vi "PECT - Scan_time gate_counter - 2.vi"() -> ()   [LabVIEW 2012]
uses:
  <vilib>/DAQmx/read.llb/DAQmx Read (Counter U32 1Chan 1Samp).vi
  <vilib>/DAQmx/read.llb/DAQmx Read (Analog 1D DBL 1Chan NSamp).vi
  <vilib>/DAQmx/read.llb/DAQmx Read (Analog Wfm 1Chan NSamp).vi
  <vilib>/Instr/_visa.llb/VISA Configure Serial Port (Instr).vi
  <vilib>/DAQmx/create/channels.llb/DAQmx Create Channel (AI-Voltage-Basic).vi
  <vilib>/DAQmx/create/channels.llb/DAQmx Create Channel (CI-Count Edges).vi
  <vilib>/DAQmx/configure/timing.llb/DAQmx Timing (Sample Clock).vi
  <vilib>/DAQmx/configure/task.llb/DAQmx Configure Logging (TDMS).vi
  <vilib>/DAQmx/configure/trigger.llb/DAQmx Start Trigger (Digital Edge).vi
  <vilib>/DAQmx/miscellaneous.llb/DAQmx Fill In Error Info.vi
  <vilib>/express/express analysis/Spectral/Block/exnSpectralBlock spectral measurements PSD poly.vi
  <vilib>/express/express analysis/Spectral/Block/exnSpectralBlock spectral measurements PSD WFM.vi
  <vilib>/express/express analysis/Spectral/XNode/ExpressSpectralMeasurementsBlockNode.xnode
  <resource>/objmgr/daqmx.rc
  <vilib>/measure/NI_MABase.lvlib
  <vilib>/Platform/NI_3dgraph.lvlib
  <vilib>/DAQmx/write.llb/DAQmx Write (Analog 1D Wfm NChan NSamp).vi
  Global_data.vi
  <vilib>/DAQmx/create/channels.llb/DAQmx Create Channel (AO-Voltage-Basic).vi
  <vilib>/DAQmx/write.llb/DAQmx Write (Analog Wfm 1Chan NSamp).vi
panel:
  in  "Repair Line Col":bool
  in  "Repair Line Row":bool
  in  "Line Col":dbl=167.0
  in  "Line Row":dbl
  in  "Filter":bool caption="Scan"
  in  "low cutoff freq: fl":dbl=40.0 format="%0.2f"
  in  "Backindex":i32
  in  "Backdata":bool caption="Scan"
  in  "ColorMapAutoScale":bool=TRUE
  in  "Min":dbl=-0.8
  in  "Max":dbl=0.6
  in  "Inverse":bool caption="Scan"
  in  "Odd":bool caption="Scan"
  in  "DiffY":bool caption="Scan"
  in  "DiffX":bool caption="Scan"
  out "Completed":bool
  out "Motor Pulse Count":i32
  in  "Counter Pulse from Motor":tag="Dev6/ctr0"
  in  "Input Counter Terminal":tag="PFI8"
  in  "Open tdms":bool
  in  "Pulse generator":T1={"Waveform Type"=2, "Amplitude"=10.0, "Frequency"=1000.0} {"Frequency" format="%0.2p"; "Amplitude" format="%0.2p"; "Waveform Type" items=["Sine Wave", "Triangle Wave", "Square Wave", "Sawtooth Wave"]}
  out "Cur. X":dbl format="%#_4g"
  out "Old X":dbl
  out "Cur. Y":dbl format="%#_4g"
  out "Old.Y":dbl
  out "Compare X":dbl
  out "compareY":dbl
  out "y >= 0":bool
  out "x >= 0":bool
  out "move X":dbl
  out "move Y":dbl
  out "deltaY":dbl
  out "delta X":dbl
  in  "Move Distance":dbl=5.0
  in  "Emergency Stop":bool
  in  "Stop 3":bool
  in  "Home Y":bool
  in  "Home X":bool
  in  "Back":bool
  in  "Front":bool
  in  "Left":bool
  in  "Right":bool
  in  "Stop Scan":bool
  out "Start Pos. X":dbl=-22.5 format="%#.4f"
  out "Start. Pos.Y":dbl=18.8 format="%#.4f"
  out "열거형":T2(ring)
  out "숫자형":i32
  in  "Gate 2":dbl=50.0
  in  "Gate 1":dbl
  out "No.data":i32
  in  "Save Scan mode":bool caption="Save Process"
  in  "Plot style":i32(ring)=5 items=["cwLine"=1, "cwPoint"=2, "cwLinePoint"=3, "cwHiddenLine"=4, "cwSurface"=5, "cwSurfaceLine"=6, "cwSurfaceNormal"=7, "cwContourLine"=8, "cwSurfaceContour"=9]
  in  "Stop 4":bool
  in  "ViewMode":i32(ring) items=["cwViewXYPlane", "cwViewXZPlane", "cwViewYZPlane", "cwViewUserDefined"]
  in  "Scan":bool
  in  "Open csv":bool
  in  "Tab Control 2":T3(tab)
  out "Hall sensors signal":waveform(dbl)[](graph)=[{"t0"=timestamp(3525645621.636764 s since 1904-01-01), "dt"=1.9999999999999944e-06, "Y"=array[2100 elements], "attributes"=variant("NI_ChannelName"=variant(string "Dev1/ai0"), "NI_UnitDescription"=variant(string "Volts"))}, {"t0"=timestamp(3525645621.636764 s since 1904-01-01), "dt"=1.9999999999999944e-06, "Y"=array[2100 elements], "attributes"=variant("NI_ChannelName"=variant(string "Dev1/ai0"), "NI_UnitDescription"=variant(string "Volts"))}]
  out "Feature Extraction":dbl(graph)=0.021153968958947764
  out "Waveform Graph 2":waveform(dbl)(graph)
  out "Power spectral density":cluster{"f0":dbl, "df":dbl, "magnitude":dbl[]}[](graph)=[{"f0"=0.0, "df"=238.09523809523876, "magnitude"=[-25.4340272409559, -28.495970805276507, -69.09064054555873, -79.11355871279994, -75.69366097931027, -84.18131507822396, -80.50168881348966, -82.72314293089615, -87.19630499623688, -82.83568021481967, -89.95290866002237, -85.90392585035596, -87.41269111550386, -91.40893948681482, -86.69370819914215, -93.36336146616782, -89.019380476413, -89.73232030153878, -94.58261196624535, -89.16287927388944, -94.965890302584, -91.86846413178648, -91.95327957161693, -97.62687167891286, -91.59993648735762, -97.30685711015555, -93.8350762480425, -93.27921214218685, -99.59438563802183, -93.1824258709588, -98.3113125531512, -95.45425138584356, -94.39327135467576, -100.65352961491782, -94.55889081970952, -99.40788907105079, -97.93617495318924, -96.19517579047603, -103.97036797797732, -96.40295202889732, -99.7036956909043, -99.48760137175819, -97.46192979187015, -106.29271483151813, -97.51447379981207, -99.86179280251669, -100.43811038443037, -97.59011642740829, -105.58363666166275, -99.01126121197593, -101.01575323613292, -101.90167607549864, -98.61952569586691, -106.73670466995647, -99.29976101634999, -101.54959604687718, -105.17330050767885, -100.09392305285375, -109.78264848704497, -100.98914236173123, -101.81665207962125, -105.42358374403365, -99.82880728595141, -107.07330885402075, -101.07712607444097, -101.03780825357597, -107.32811151840846, -101.221643458408, -105.63776326231454, -101.8420593566944, -101.80081629073969, -107.47915505307212, -101.12986632760553, -106.84901404755908, -102.73715610491038, -101.51552854007832, -107.28771371003282, -101.3928633472346, -107.44515355816633, -104.89304864643535, -103.1455098860718, -110.19910428997925, -102.73063833081197, -107.57101838377707, -104.90574568581201, -103.72599931018533, -109.97178587260123, -103.24611921258705, -108.36098023558972, -106.6408311450923, -104.73569536588386, -116.21683530762306, -105.02627439976544, -107.15856030450797, -109.81191038702062, -105.53476822084077, -119.10077766590356, -105.31867536160968, -106.9718410299748, -108.34458911268797, -104.70307996109247, -114.76704583683203, -106.29948298493936, -108.55077108437321, -112.16618350190343, -105.98453547558171, -114.68576835450673, -107.50968901677987, -107.89174277914348, -111.59875709602721, -106.69368240333122, -114.93273233954758, -105.23904516482949, -106.00272331017348, -110.36103151258544, -104.93177986717492, -110.8835476773746, -106.69346348818806, -106.66103973993782, -119.11729839814336, -108.06338160849775, -114.5879267769655, -108.59816838472844, -107.53189260743514, -114.07390818184973, -106.70996756049796, -113.27381274118753, -109.50270539577696, -107.37282420343303, -113.4779718725949, -106.04267666963091, -111.30294425571472, -112.46717993668915, -109.13164915488709, -116.65287200885172, -107.03002573045511, -110.21479040603631, -112.476075561056, -106.97710947409149, -119.42145279296255, -108.3200486628316, -110.46641858585929, -117.16650627564961, -109.73297826697552, -120.31689830731365, -107.19513745371916, -110.66663569403087, -113.30365980039964, -110.01971553524372, -123.68660617105166, -110.8171755739396, -111.11382172813546, -117.76239209582961, -109.49899370205401, -115.22252846498625, -111.1932077339224, -112.38235939086871, -118.22207022901702, -110.6546796895719, -116.97450780644367, -110.82401674194465, -111.96705198878843, -118.28092956599232, -110.5621503678909, -121.25720613496851, -111.98371482341479, -113.27928013246557, -111.96833712758355, -108.56859286664552, -120.32790468431601, -110.82699792221703, -110.79062667340345, -122.65756767769517, -110.48843456045427, -116.8782055296399, -115.43719816168479, -114.47619780315773, -121.42183196132746, -111.60631415727042, -120.68077308056417, -109.35478690141552, -109.03210709352732, -120.6260555904793, -109.47936424950136, -113.33719701518146, -112.88325992990137, -110.99901978536154, -123.19636626521421, -109.09861317900774, -113.33125158106256, -115.35673297389727, -112.77249677632989, -124.61163141716472, -114.68140920359865, -121.89642913325117, -115.47413298424323, -112.82196063671608, -127.87542521315149, -111.54178118788309, -113.6448752704395, -120.76569423868874, -112.98651214877823, -123.18868565400437, -115.41399838634062, -115.46853076016815, -116.40989072804102, -110.69611347288615, -132.23164080331392, -114.76376391429793, -121.7246597336247, -117.46893009589195, -114.01899156779395, -125.22079066032327, -114.59524199183258, -114.50034890537415, -122.9532092227648, -113.72727798159212, -125.65163915514907, -113.4793801211504, -110.4090756414644, -125.63592649005872, -114.22938378193007, -116.74947251106808, -121.60535557984142, -116.79385283402802, -122.44667696630361, -113.43873413563811, -123.28159708694415, -113.92892974938164, -114.01193823589753, -121.62751955742443, -118.76839573694522, -125.52998605097204, -115.19609643487229, -117.49409595176479, -117.08423885198002, -119.48314867245172, -125.01675515413412, -117.92668164142911, -115.55962389856793, -125.63488616674975, -119.11862859365166, -114.78860770332909, -117.18339781294443, -111.18063004722558, -118.31775966044624, -111.6867367949252, -114.57226159377, -119.36541212960576, -113.90245139442648, -132.46343443313128, -120.1282759002165, -121.05279009698619, -118.9115822659523, -121.23280439248342, -116.31914159559688, -127.38829313950257, -117.34673005740623, -115.95249861902771, -114.9301657394146, -123.22361802797445, -110.83274939062106, -116.16624248562111, -116.76753364192771, -113.94454545069023, -122.95736945775944, -118.66755800656253, -129.1462641201204, -116.6351050110328, -117.22529407303742, -123.80212197360244, -115.89792176423389, -114.25823938606595, -125.60467961977515, -114.59958849364433, -121.70071005514421, -118.25968972451209, -114.69929400946009, -123.88209034116528, -115.03869272537257, -117.52034211782204, -115.27990843516797, -117.85366603932033, -125.16865559622727, -118.21960424638507, -119.69008755413566, -117.24640963460672, -114.32867295013791, -119.1576982419508, -122.85495988425586, -116.3373010103401, -114.53730203699834, -115.67017599990201, -127.144321037601, -115.73849102686786, -117.7626163106355, -119.7346592991025, -117.41317517684553, -125.0417974461613, -114.5488949833583, -116.59812516173781, -119.91064563147799, -115.27933218667663, -122.09990513751134, -120.95678574143693, -123.25641714743752, -112.5173710452192, -113.53735878806998, -129.23914933506734, -116.27157269711533, -148.4020512032711, -118.84888216023774, -123.82550527215588, -116.87770979616658, -111.32191810025745, -124.32675905891588, -114.37182733794062, -121.10713785851372, -122.59698730059695, -116.38346694563282, -121.69144349152856, -119.00883142493832, -110.81886738196273, -120.7909830607913, -115.01780448665316, -114.52055121633796, -132.6824191654361, -116.330695115645, -126.4664151018508, -118.32717907779282, -118.7288071595281, -120.42749846140066, -112.53185615773879, -124.26026008984286, -114.24089252048742, -120.00368190003405, -114.71738500842926, -112.92262025927133, -129.21127897188563, -113.5947811765517, -117.80802009651353, -117.0133790103226, -112.19210322760304, -118.17549968071762, -119.3256187825503, -118.84981507334446, -121.39118969751144, -114.64543555194373, -119.84814933224528, -114.09123407848944, -116.22899352170892, -116.41650104077173, -113.70057202673476, -124.52773908304957, -114.87372641784933, -116.11651108221098, -121.68680962246994, -115.78306007961302, -122.22621008657796, -118.81157995182392, -113.9402115821658, -132.636729517989, -114.49554876936634, -119.50980190398928, -123.27410972236837, -118.52851881066383, -122.25212982572599, -117.13947036230024, -120.85005588797962, -118.41526503460501, -117.61788553858068, -126.3872056783977, -114.98198608543298, -119.7789938911847, -120.84873579392627, -114.38831474301695, -153.35954756825245, -113.19505610638078, -114.17454820985151, -127.41069917723112, -114.92677241657191, -125.49053973810628, -113.36382196587914, -119.96785250843519, -122.47388530423243, -116.38671253508838, -120.0905790211523, -119.83326265062107, -117.88168146696918, -122.3132169880757, -115.87324909105399, -125.92003267803432, -113.96860176867415, -114.49156118371398, -127.52634390035722, -115.05967156528004, -126.82020221981517, -117.93643187259194, -116.51163213641807, -119.47551219110167, -119.55225172256931, -116.9512257852571, -122.23153124485954, -120.8368476753637, -121.48473913072222, -115.83122660909913, -135.74260014140523, -116.58358375805423, -118.15236945484727, -119.06674062398864, -115.7844834762477, -125.06111738611818, -114.7801535050972, -115.2696605691888, -123.98656374010793, -119.29025555731172, -118.29146803784099, -119.55696172158135, -118.06884171238352, -127.81587648134607, -120.41730580797976, -123.49626136731604, -112.2147141798107, -116.22555232584983, -132.79419178871254, -119.66964883124663, -117.20946469243259, -118.20939292735417, -115.6951914646649, -129.64892855822356, -114.27056999288617, -120.31005512957381, -117.41846777372632, -115.50158386260813, -124.69777160737624, -115.2892897247205, -123.61522771666871, -113.75248734362687, -113.22999749252833, -129.3490509395313, -116.88137735661701, -116.94110280242681, -119.50244079984806, -119.30521139999144, -128.17199984115797, -118.06736594940236, -116.05331575995922, -121.29670750650897, -116.1140297602044, -125.090619084802, -121.41807296062154, -120.01332757902264, -120.54914530643151, -116.49738633175463, -122.32551291835904, -118.3190808346865, -118.92638453656723, -122.48819531011718, -117.01021725424317, -120.98896352560598, -117.23831688685218, -121.27915259197124, -121.20017251921661, -117.6155648860373, -120.91300272912063, -117.94438460863424, -115.94437430101533, -123.35904829443987, -117.74011174503076, -121.54935745388448, -120.82564553545025, -121.98951430455743, -120.24858103448778, -116.44403527138395, -112.79571494351876, -112.42801913096545, -110.1697573019791, -115.34500457736401, -119.81921052956707, -129.82600951154313, -115.5862301263047, -112.59292882433087, -120.79009137478283, -131.32849293387295, -113.61194478398238, -123.48568856527031, -119.17507777781304, -123.09261867490484, -116.97755217417308, -123.94453461434183, -116.58080525616379, -119.64289646280756, -122.90202645580743, -126.66219093058154, -121.95048829056148, -115.72578023509817, -116.70117814464484, -121.91050280869723, -118.25299095698178, -116.45905559047064, -132.57794493731578, -121.65327820443292, -120.9816664775787, -117.17270262269045, -120.27433984830965, -125.89418976028173, -119.09563505847817, -126.9693215534833, -113.17465524665704, -118.98702092883116, -119.83822568580342, -120.45832738089722, -120.67735960513633, -127.38676010839353, -127.65777338183055, -118.37446329057411, -115.61355494839711, -119.94568688114103, -116.06619937633681, -126.348857777089, -118.92850079147068, -119.5416617639739, -132.47075644221843, -118.08809356028496, -123.16186463092723, -121.51579486791232, -122.88983670053283, -129.5195538417256, -120.4730389608841, -132.16486858341602, -122.34690358436781, -120.71922104337597, -114.29260860841114, -117.67902631803368, -124.7040155514909, -123.51274592117205, -120.02297921674332, -136.54655493811157, -120.45629227407751, -119.06410204276258, -127.91681714792554, -122.82090055753153, -125.16838176650813, -121.79565386970478, -119.79607311590995, -126.54861375039647, -121.59135878113302, -132.8348640697562, -118.1305434733294, -120.46070148841905, -122.69571910896963, -117.6534954653865, -124.15742546824006, -120.73646926947502, -124.82696993800742, -124.513836786494, -123.15395713389651, -124.62395468806395, -117.21365768658171, -119.32635871968456, -121.48532284413152, -119.38242892643675, -126.25575652510352, -123.27133124029851, -117.58533922728374, -118.17710108929799, -114.99496360200965, -117.77133194647278, -111.34898201101595, -111.50817058307922, -119.0703124690998, -127.70676079885351, -121.8704969141074, -125.93154214283446, -118.65628450081473, -122.47918878348962, -117.9651589546518, -126.13560583004508, -122.42294805637847, -133.924453763793, -117.2082573038767, -117.6525335446734, -122.92077297426977, -122.04624645756786, -116.43289028226238, -117.93180959338378, -129.02356734231915, -117.95493621286326, -120.7555929766252, -120.76782849311112, -123.06287498470708, -117.83798593857965, -123.43423215434719, -120.15190119516652, -120.48240443128407, -143.29738987393452, -123.46572247444769, -120.89055325172792, -125.66715973809033, -118.26887578998644, -117.01836200028421, -121.33021830755509, -119.68846363313813, -122.60689066103069, -116.26858138914181, -119.59360791972998, -122.94866175463353, -114.174409515556, -118.00516930888391, -121.56978543579633, -135.87799017759036, -117.50816594504829, -122.82539428457626, -123.82103443155845, -124.77975840345442, -121.13340798086698, -120.93607435603558, -133.15787160745222, -120.70545628137863, -125.02155972441679, -122.04666465472178, -118.01234649746348, -127.88767491042842, -119.02096620167217, -120.16031065152875, -122.25406107859625, -121.72733059051095, -120.61357375519918, -118.63962847172827, -134.3857741605498, -116.3600853185034, -117.26695700691671, -119.9176982185873, -113.45576465218444, -126.69779573632724, -114.39554522802246, -116.8457146515868, -116.34219889483086, -119.30011291548334, -120.01163291843496, -114.29497178248809, -127.65687642749229, -119.58556923753022, -129.8593054181261, -122.2353645100479, -120.79536520223796, -119.83284028355028, -117.7991246185715, -128.390292904734, -119.78079925213122, -125.478913448993, -113.89747777944768, -112.66620124153357, -124.3475049842711, -120.85847303094337, -132.91807981902295, -119.523494985723, -116.65149909866443, -119.73287290436721, -127.63237851524192, -127.23413304048789, -120.87585453904362, -121.08540368080186, -134.91071939669257, -117.75375801669338, -117.2683014590723, -120.9739099492833, -118.23809733632451, -120.94065804928206, -123.88077510875804, -118.13812819300607, -122.60294123365466, -126.97075898006995, -120.18754789731035, -124.71238663441227, -120.55456557278582, -130.94599087480253, -111.18288669417035, -112.27708791831247, -126.0512034600378, -117.41881712783596, -128.20553880273903, -117.29482600885808, -118.2045526390752, -127.81966672699878, -117.03716165902529, -115.46711739757512, -117.15363929234843, -121.87599671671335, -121.19736800869221, -126.5301786755875, -131.20754947382918, -124.40138004810741, -129.0562496906515, -121.06816554587536, -121.01023627802867, -138.6137911215848, -120.12495002524031, -121.38510517514229, -122.79804220535513, -116.97501378195477, -118.82011581137473, -114.0229185604644, -119.54287501990726, -114.64474566771625, -117.76935669872461, -123.81082574158907, -118.51678358865587, -128.9664755188374, -123.45357998434133, -122.74888841574231, -120.74640581234044, -126.956344345126, -119.95682140104577, -118.8873101779055, -124.41062359284174, -128.97304498664363, -123.86287113204068, -127.30257087528216, -120.61364220528216, -114.45119129304715, -119.68384044686806, -131.29639185291157, -122.31250766293485, -119.57420865241102, -124.74014026002448, -124.87593035709094, -118.4566565612952, -123.76236085976001, -120.84780538841838, -117.68987599773281, -135.06195695255914, -122.56143585795171, -129.04610316842883, -118.32313199570537, -117.77093802786419, -124.46572845786741, -129.1123298336903, -120.88470269965448, -116.69988985752187, -116.84054667499878, -133.76883696987278, -122.32434984927302, -124.98940594457933, -122.56515592789917, -118.31562562243366, -133.97049179545627, -122.33220627999802, -131.16753675316977, -124.69828063969263, -116.37621154460467, -126.1833423168025, -129.62937634161355, -118.46241371150788, -117.52851478852457, -125.32425037236442, -119.0327364293772, -124.2861355894013, -123.24573502278234, -125.52155812053758, -113.75743410709823, -114.79513162658353, -128.58142362588052, -122.48277095196701, -118.94747544412269, -123.86988127835491, -124.78140456983323, -121.53998481875398, -116.01432822539552, -119.20174681160661, -122.75167725800814, -120.58657749420254, -118.51141061842183, -119.24457006171983, -131.43641234223372, -116.00759139055087, -121.24442216102587, -123.29371279953725, -117.608355420454, -116.33684374617326, -118.06291688281922, -121.88761866022774, -121.54820313120047, -119.5051369873635, -126.56611158390913, -118.84012713615805, -121.09285296522563, -124.67955377692547, -147.31451139022337, -116.80660421066897, -114.8367853755961, -120.41026468628925, -123.65666101895222, -119.64837119787269, -116.77480172559095, -116.54263359173909, -124.75286620868079, -117.33721912698883, -116.51795620907136, -118.50086748176733, -128.10381328920522, -122.78098994574157, -120.24716756092855, -119.52743204722819, -115.00407387659232, -108.2853711552629, -108.61086943894702, -119.6228894146785, -124.11132022420912, -125.6202218409766, -123.1749360787656, -118.1971196161698, -123.95075368058998, -121.72140109898365, -123.27106899042522, -123.73035629887062, -121.24369679109273, -121.07381526465288, -113.13965659723667, -118.330755475899, -118.40249076804484, -111.59630598649044, -116.1569506845575, -125.67326089915758, -125.85723567111906, -119.24293277595024, -117.87067617433537, -120.70936924059559, -131.8090588468898, -132.98711569625004, -123.63274249467587, -122.75476917502559, -126.12873814250243, -120.53144270605179, -129.07030822919336, -122.7889410422919, -124.35405971166259, -119.63968579420454, -139.0154441054289, -129.47962001806934, -121.86548015410847, -128.6818469257012, -121.40195873232601, -138.64231053781285, -124.22025721762265, -124.06073958736941, -126.71929802352521, -131.7498459276443, -120.68144109742178, -122.6325588818875, -126.80796617875095, -124.92487955227033, -136.94498040498806, -124.26704334219014, -123.21376211221711, -140.25352033075964, -129.53222319772195, -122.58541579060463, -122.1996729592375, -125.66642108013673, -125.66310429236694, -120.09682773706965, -125.27326633941439, -121.55721878725502, -121.22507119941083, -121.53716878624485, -136.20685498111987, -128.15260146013156, -120.03473972471616, -124.60755958763912, -124.73082500077143, -123.93425949983688, -131.04483249265184, -121.7957035014449, -127.09321441816094, -133.6144579272493, -124.69014595896968, -130.4902091211609, -121.18031440773905, -128.00033943961677, -125.88991118115149, -118.865310745079, -123.69668867733147, -117.98756965862728, -114.40013091842827, -118.28685032521078, -122.23464196869948, -124.8440422629961, -129.66281606870848, -119.440534215621, -124.54391783563877, -124.93447967158188, -121.7258558761523, -122.28817885403082, -127.06889620458577, -128.92172974939206, -120.62932166634072, -126.06847321900452, -123.31471168429935, -121.80350826545656, -129.2574604322076, -125.67225933193998, -125.7801671825605, -129.53804733161627, -119.56756644124712, -128.82490314699373, -124.7689736295626, -120.50019729114693, -124.50603158563972, -122.8120627011088, -125.60528875555717, -123.8817354922713, -124.05570537836674, -120.94568834491936, -118.06056028605255, -124.24390361274648, -125.5716703018188, -127.71949519914061, -130.7001652968252, -126.27701412017494, -133.76810134709916, -128.4738939614179, -120.302550881701, -118.91298143662928, -124.9077318110765, -127.16253699189492, -118.11405934812818, -117.52028071290711, -140.95620572748925, -123.61977932545628, -131.0334379970501, -125.88948384968432, -127.81552331993379, -121.92316280719056, -119.05911238768732, -126.83773251459189, -123.52627415002164, -120.8779561023192, -123.66683567603742, -131.64300993967345, -123.62895847772963, -116.89792951363142, -120.1068259250195, -117.92484706459337, -115.58208487778379, -120.76803581628594, -123.95408562090736, -122.79456549632754, -134.5305398779298, -123.57040300991032, -128.40634159414552, -123.70102187824159, -118.24970739397313, -119.66483900349026, -127.78024313111393, -120.3547204111785, -125.49305364308705, -119.49505591004302, -120.50920386196539, -119.03509516851003, -114.24667300009652, -121.60538636584391, -119.95304417598024, -122.24585853682832, -128.63653016912684, -116.04810628805795, -121.94159862131235, -122.59928204398939, -121.4532410501923, -128.6511474663462, -130.83715595958148, -121.71998300574741, -116.91426629511156, -113.587592058512, -115.59736707638731, -124.65300822631244, -133.32538684258748, -124.02289142873636, -121.54278890993639, -119.02596809402394, -108.90572887117857, -112.14974069608851, -129.21149299565423, -118.82148342951197, -116.65510894288538, -118.39609618084175, -116.53502642884725, -122.47549439965209, -122.23125657046063, -123.68081343116663, -120.67915071600007, -123.6899360128769, -118.56721985209728, -118.36641581191942, -126.96724630704657, -119.36877661672403, -123.07698921198843, -117.80772421906035, -122.82545076270567, -118.82755071380888, -117.21030132539394, -129.760567864525, -118.0816708063509, -125.80573274113647, -121.18434666182338, -121.80987210832065, -130.99259828357094, -125.47223579895922, -123.86818606677002, -118.7118158196511, -119.27778317338742, -127.27333258839096, -119.90672352079164, -140.78772370844268, -118.08251080057329, -119.86636232122572, -118.69482489738232, -119.19106512767372, -123.70988914879189, -121.92566832147995, -123.41378261726373, -120.1715186070818, -117.9079629421116, -117.41960207545632, -123.72833996166874, -127.24377206607298, -124.99098647980887, -129.48803701799955, -129.92351350561592, -120.79284154834647, -119.29601975194524, -136.17244775530037, -126.73975437546255, -128.84068276143336, -125.66374985701982, -136.69026010435715, -125.44409235146617, -119.28138070315057, -118.65017329869724, -118.02521532826772, -122.23736063759657, -121.27846943548622, -116.69850478126861, -119.7711336696722, -123.70776561180185, -118.43344549561263, -123.92390877157247, -117.19637143066551, -117.64112988205311, -127.78399195238529]}, ...(2 in all)]
  in  "3D Surface":refnum<k7>(container)
  out "Record path":path caption="selected path"
  out "Feature extraction scan":dbl[](graph)
  in  "Tab Control":T4(tab)
  in  "Step X":dbl=0.1
  out "Move X":bool
  in  "Direction (+)":bool=TRUE
  in  "Step Y":dbl=0.1
  in  "Y-length":dbl=10.0
  in  "X-length":dbl=5.0
  in  "Save Speed":bool
  in  "Cur. Pos Y":dbl=18.8 format="%#.4f"
  in  "Cur. Pos X":dbl=-22.5 format="%#.4f"
  in  "Travel per Pulse (mm)":dbl=0.002
  in  "2 Rate":dbl=0.2
  in  "1 Rate":dbl=0.2
  in  "2 Min":dbl=1.0
  in  "1  Max":dbl=8.0
  in  "2 Max":dbl=8.0
  in  "1 Min":dbl=1.0
  in  "Parity":u16(ring) items=["None", "Odd", "Even", "Mark", "Space"]
  in  "stop bits":u16(ring)=10 items=["1.0"=10, "1.5"=15, "2.0"=20]
  in  "Data bits":u16=8 min=5 max=8 step=1
  in  "Baud Rate":u32=9600
  in  "COM Port":refnum<visa-resource-name>="COM12"
  out "No. X":i32
  out "No. Y":i32
  out "Sample per Channel AI":dbl
  out "Sample per Channel AO":dbl
  in  "Pulser Cycles":i32=10
  in  "Logging Mode":i32(ring)=10231 items=["Off"=10231, "Log and Read"=15842]
  out "Actual Sample Rate":dbl=500000.0 format="%0.2f"
  in  "Physical Channel":tag="Dev6/ai0"
  in  "Min Voltage":dbl=-10.0
  in  "Max Voltage":dbl=10.0
  in  "Terminal Configuration":i32(ring)=10083 items=["default"=-1, "RSE"=10083, "NRSE"=10078, "Differential"=10106, "Pseudodifferential"=12529]
  in  "Sample Clock Source 2":tag="OnboardClock"
  in  "Sample Rate":dbl=450000.0
  in  "TDMS File Path":path
  out "Actual Sample Rate 2":dbl=800000.0 format="%0.2f"
  in  "Physical Channel(s)":tag="Dev6/ao1"
  in  "Min Voltage 2":dbl=-10.0
  in  "Max Voltage 2":dbl=10.0
  in  "Sample Clock Source":tag="OnboardClock"
  in  "Sample Rate 2":dbl=800000.0
  in  "Offset":bool
  in  "2 Plots":bool
  in  "Edge":i32(ring)=10280 items=["Rising"=10280, "Falling"=10171]
  in  "Pulser Trigger Source":tag="/Dev6/PFI0"
  in  "Duty cycle %":dbl=50.0 format="%#.2f"
  # "Pulse Shape"
  # "Trigger Settings"
  # "Data Processing"
  # "Time gate = %T/2"
  # "Pulse"
  # "Hall Sensors Signal"
  # "Feature Extraction"
  # "Power Spectal Density"
  # "COM  Setting"
  # "Speed  Setting"
  # "Scan  Setting"
  # "Pulse  Channel"
  # "Pulse  Timming"
  # "Sensor  Channel"
  # "DAQ Timming"
  # "Logging Settings"
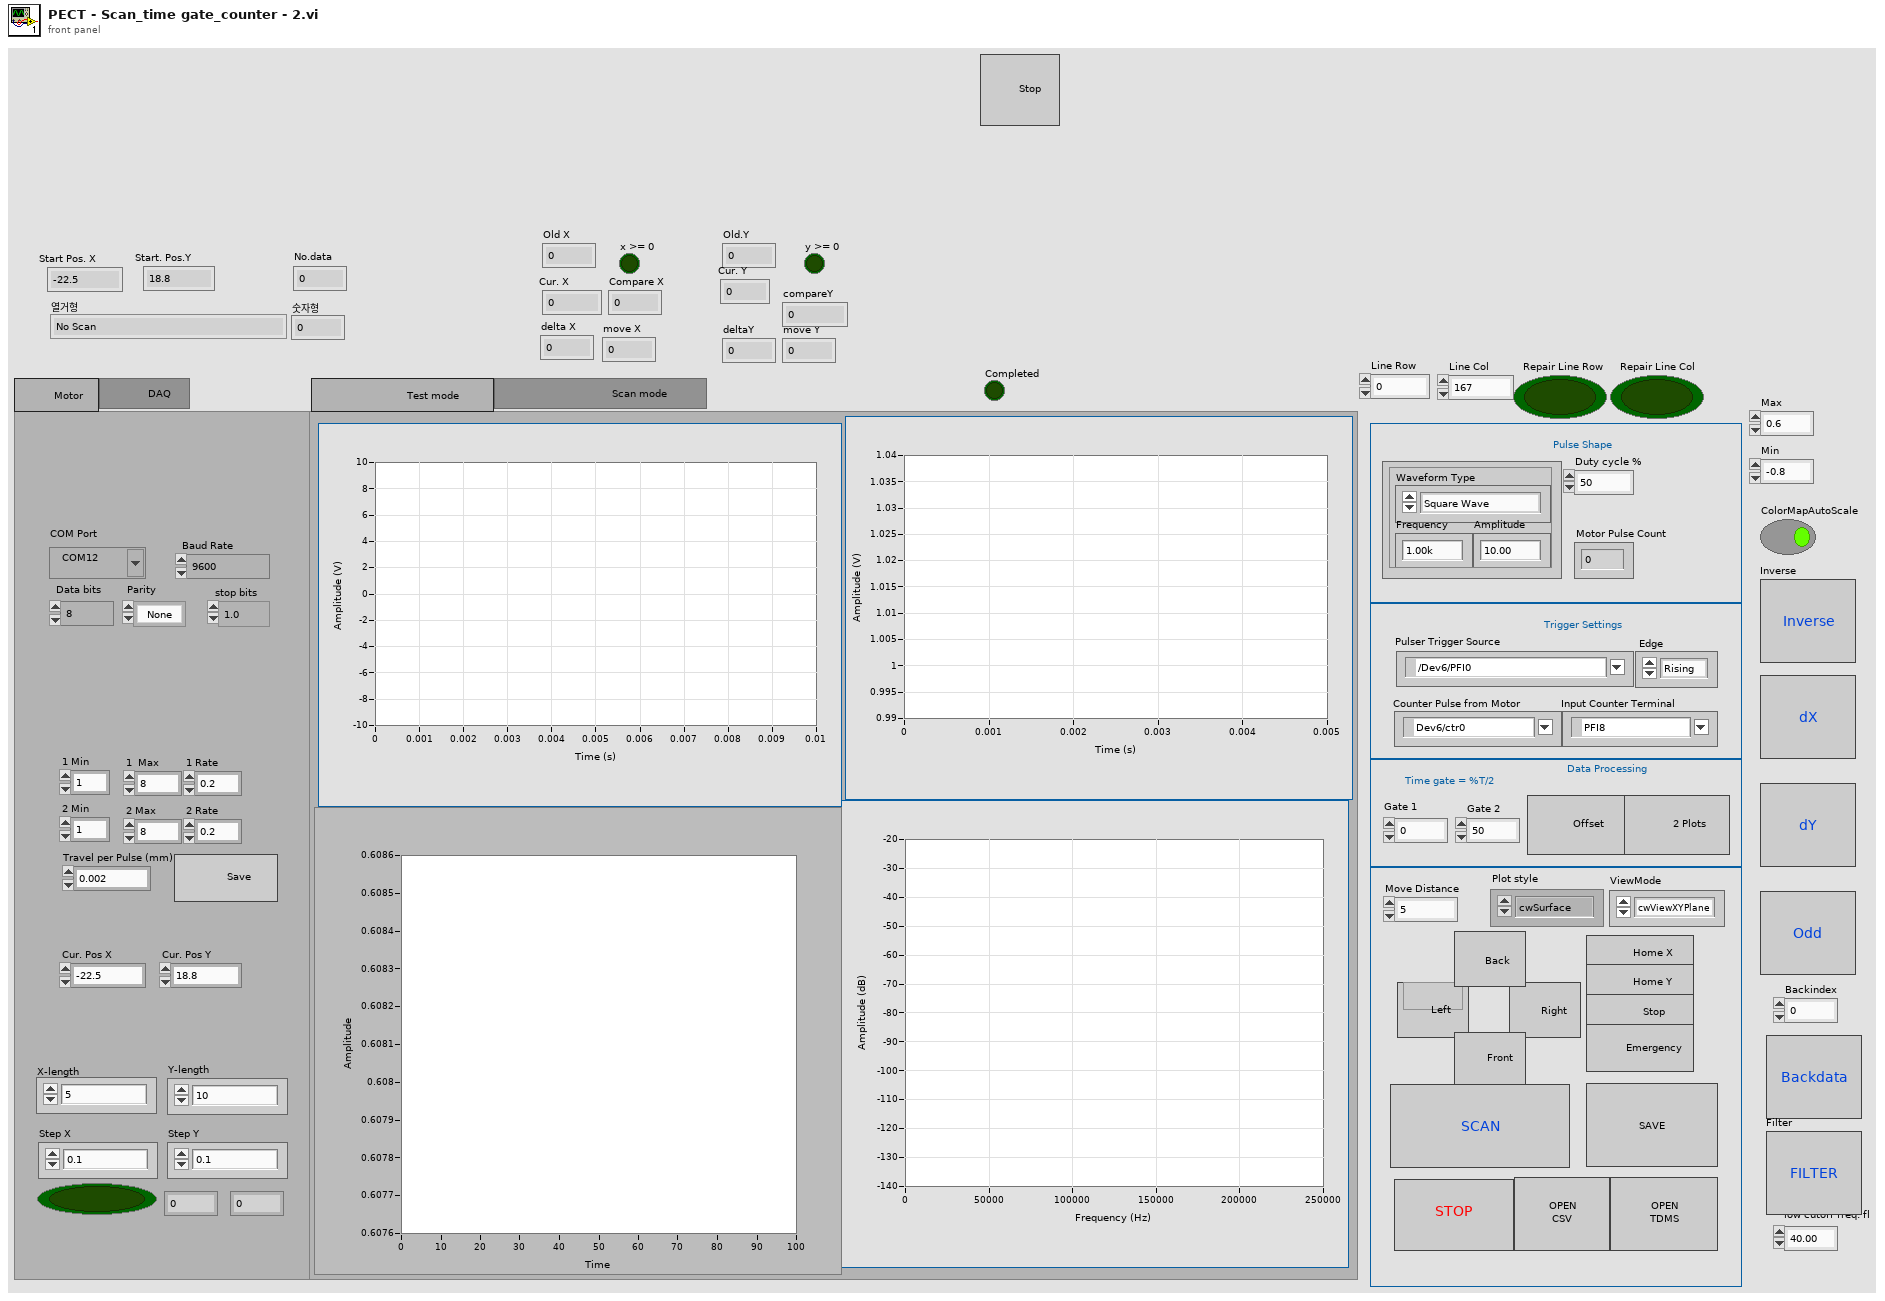
[diagram p1: front panel]
types:
  T1 = cluster{"Waveform Type":u16, "Amplitude":dbl, "Frequency":dbl}
  T2 = enum16{"No Scan", "Move X", "Wait to destination X", "Move Y", "Wait to destinatioin Y"}
  T3 = enum32{"                    Test mode                   ", "                          Scan mode                      "}
  T4 = enum32{"        Motor      ", "          DAQ        "}
  T5 = enum16{"open", "open or create", "create or replace", "create", "open (read-only)"}
  T6 = cluster{"averaging mode":u16, "weighting mode":u16, "number of averages":u32}
  T7 = cluster{"dB On (F)":bool, "unwrap phase (F)":bool, "convert to degree (F)":bool}
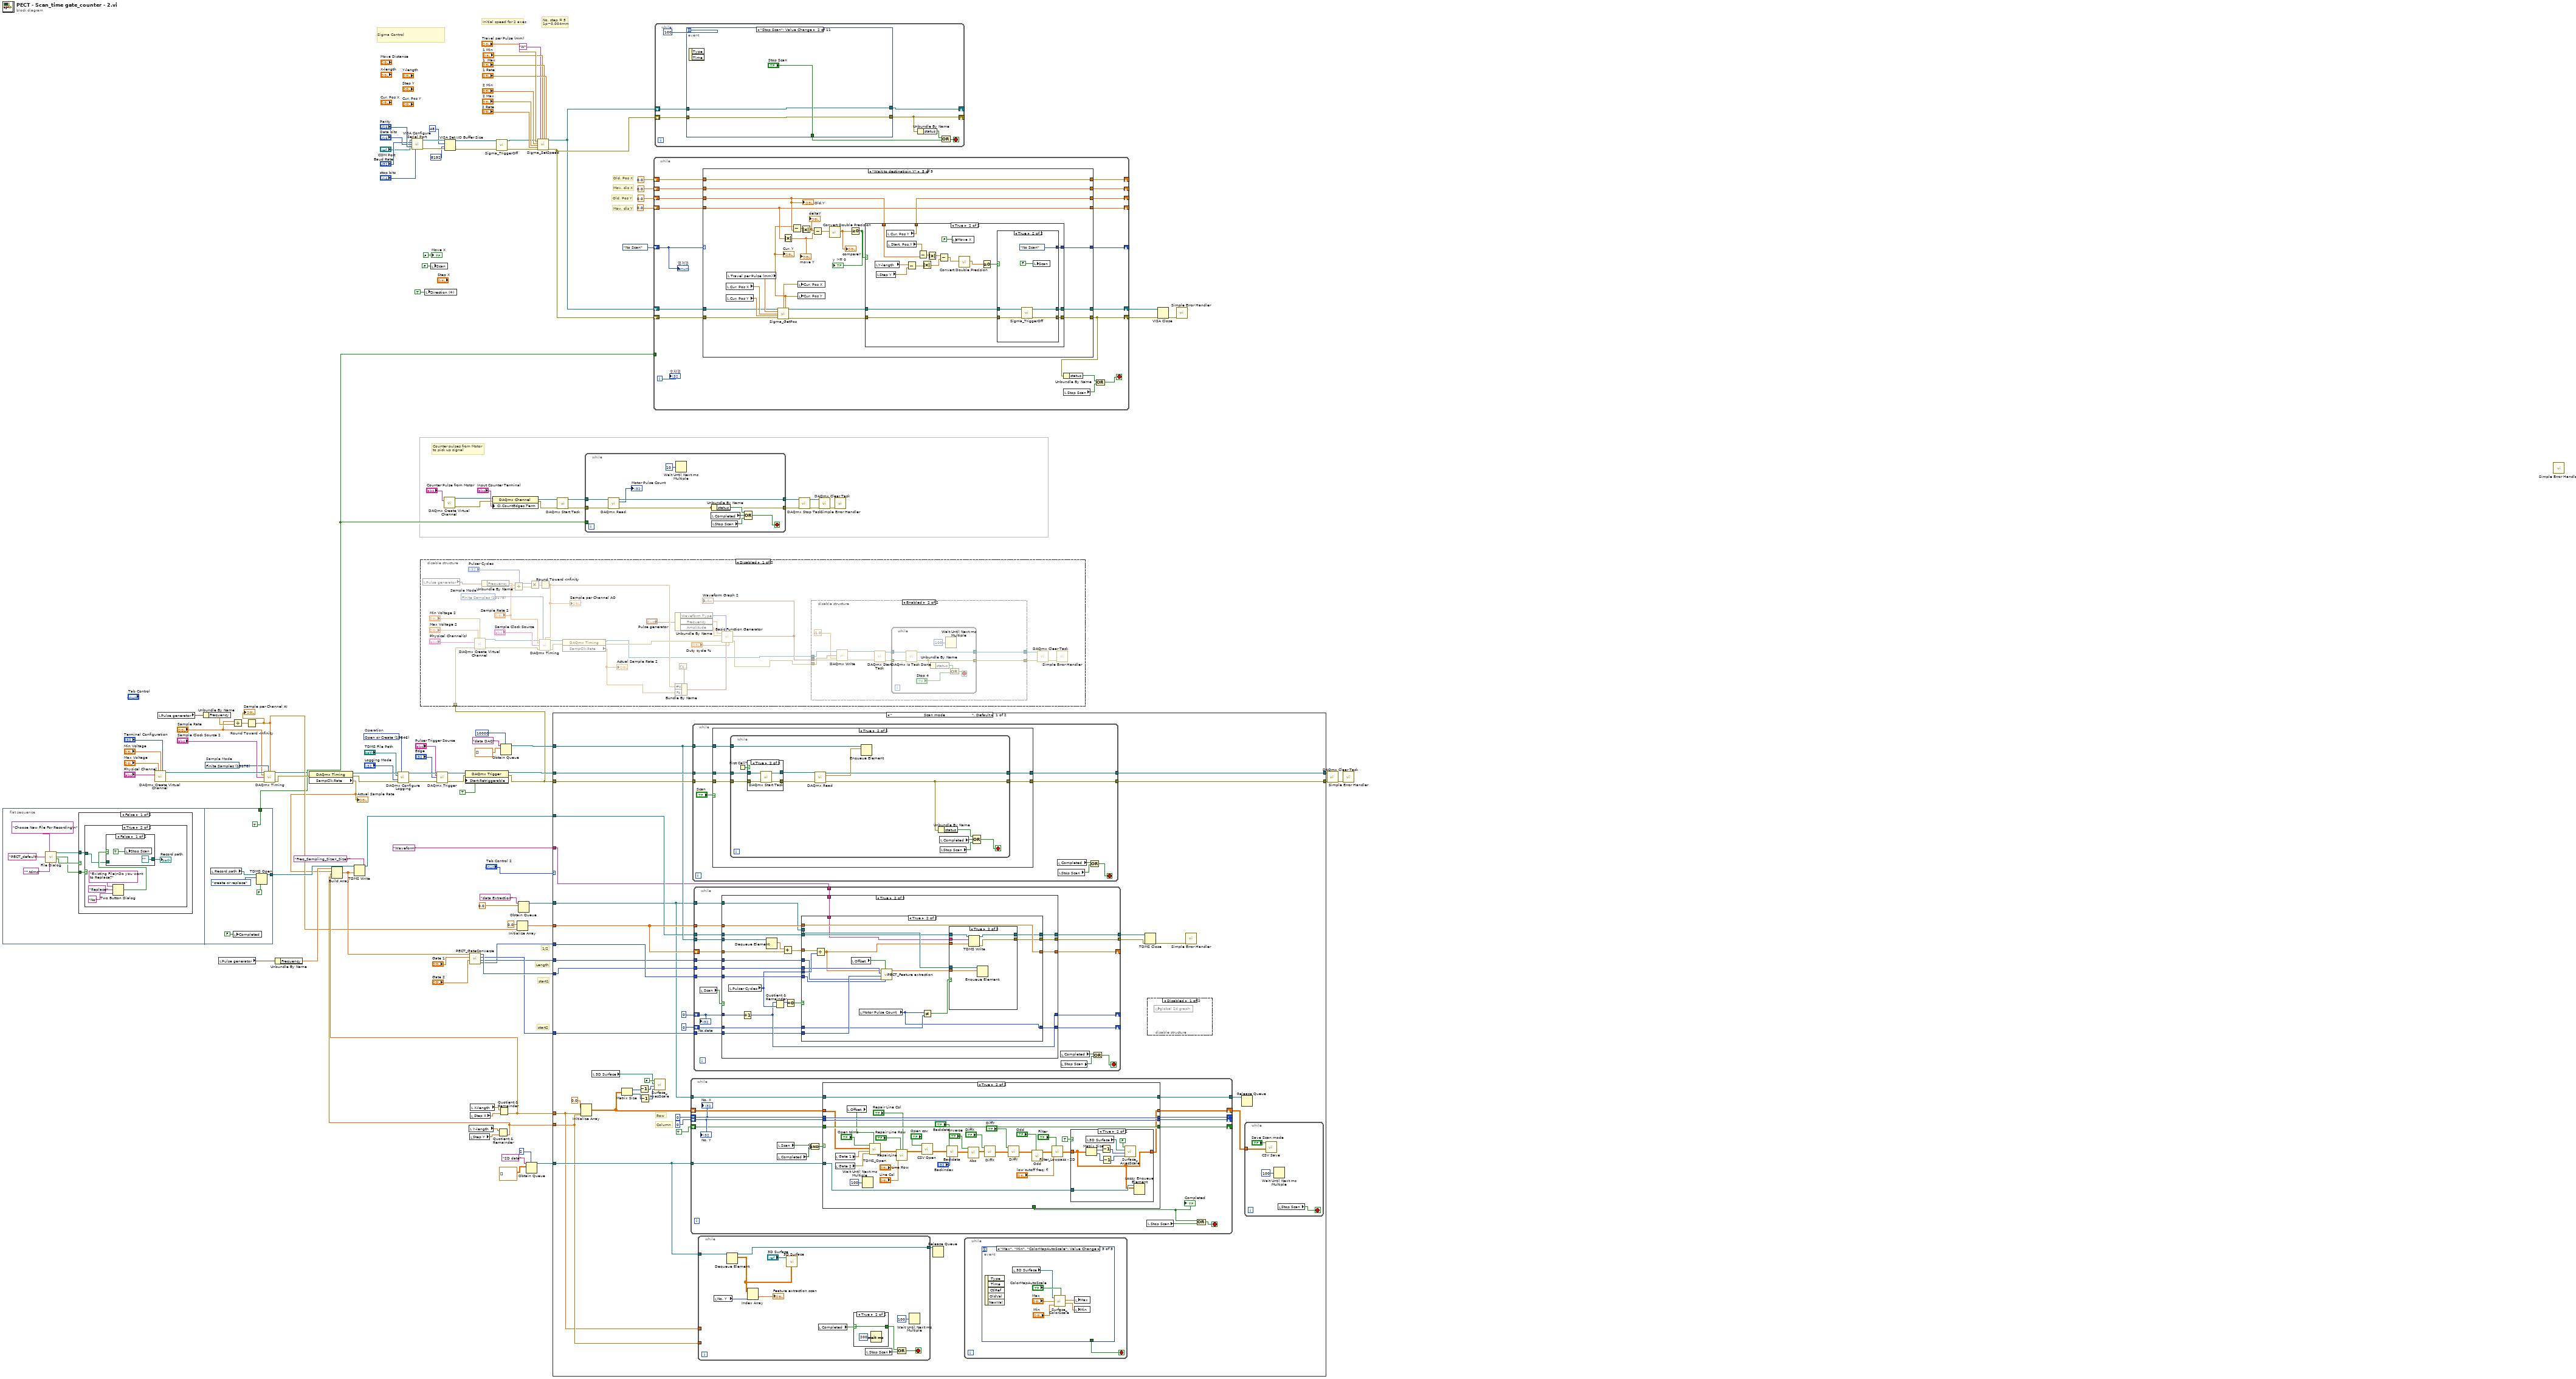
[diagram p0: block diagram]
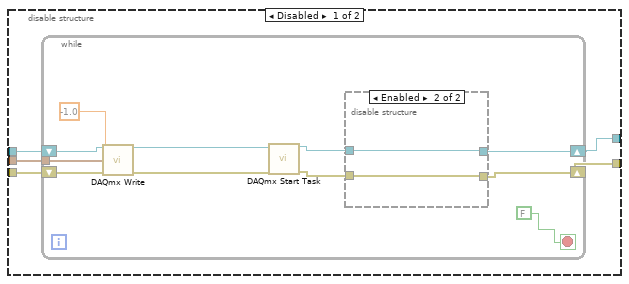
[diagram p2: hidden frame]
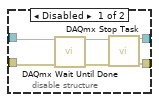
[diagram p3: hidden frame]
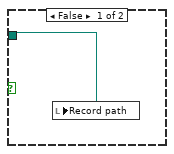
[diagram p5: hidden frame]
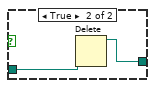
[diagram p6: hidden frame]
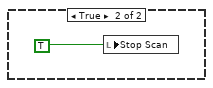
[diagram p7: hidden frame]
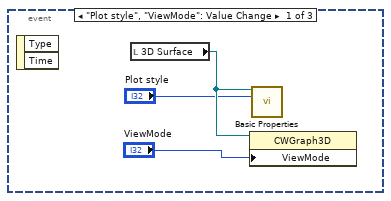
[diagram p8: hidden frame]
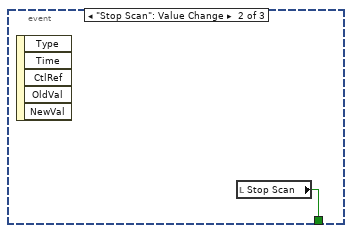
[diagram p9: hidden frame]
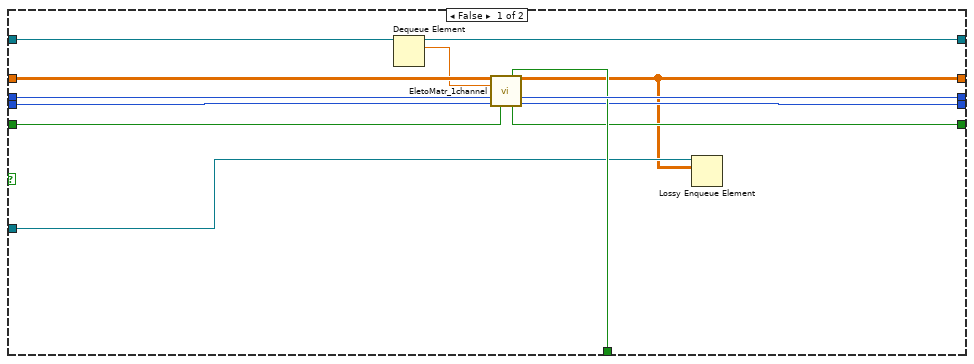
[diagram p12: hidden frame]
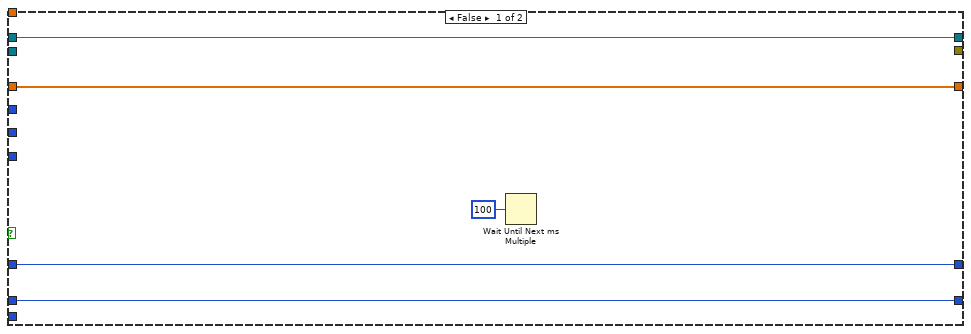
[diagram p16: hidden frame]
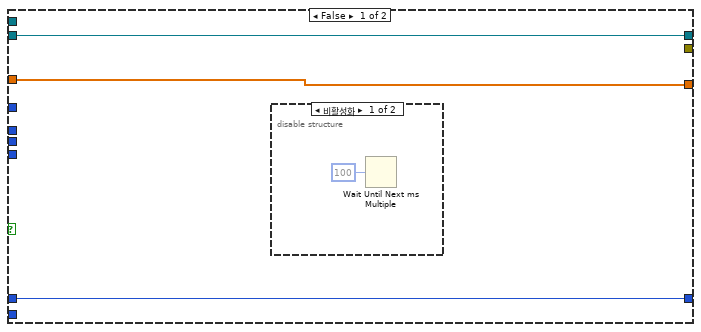
[diagram p17: hidden frame]
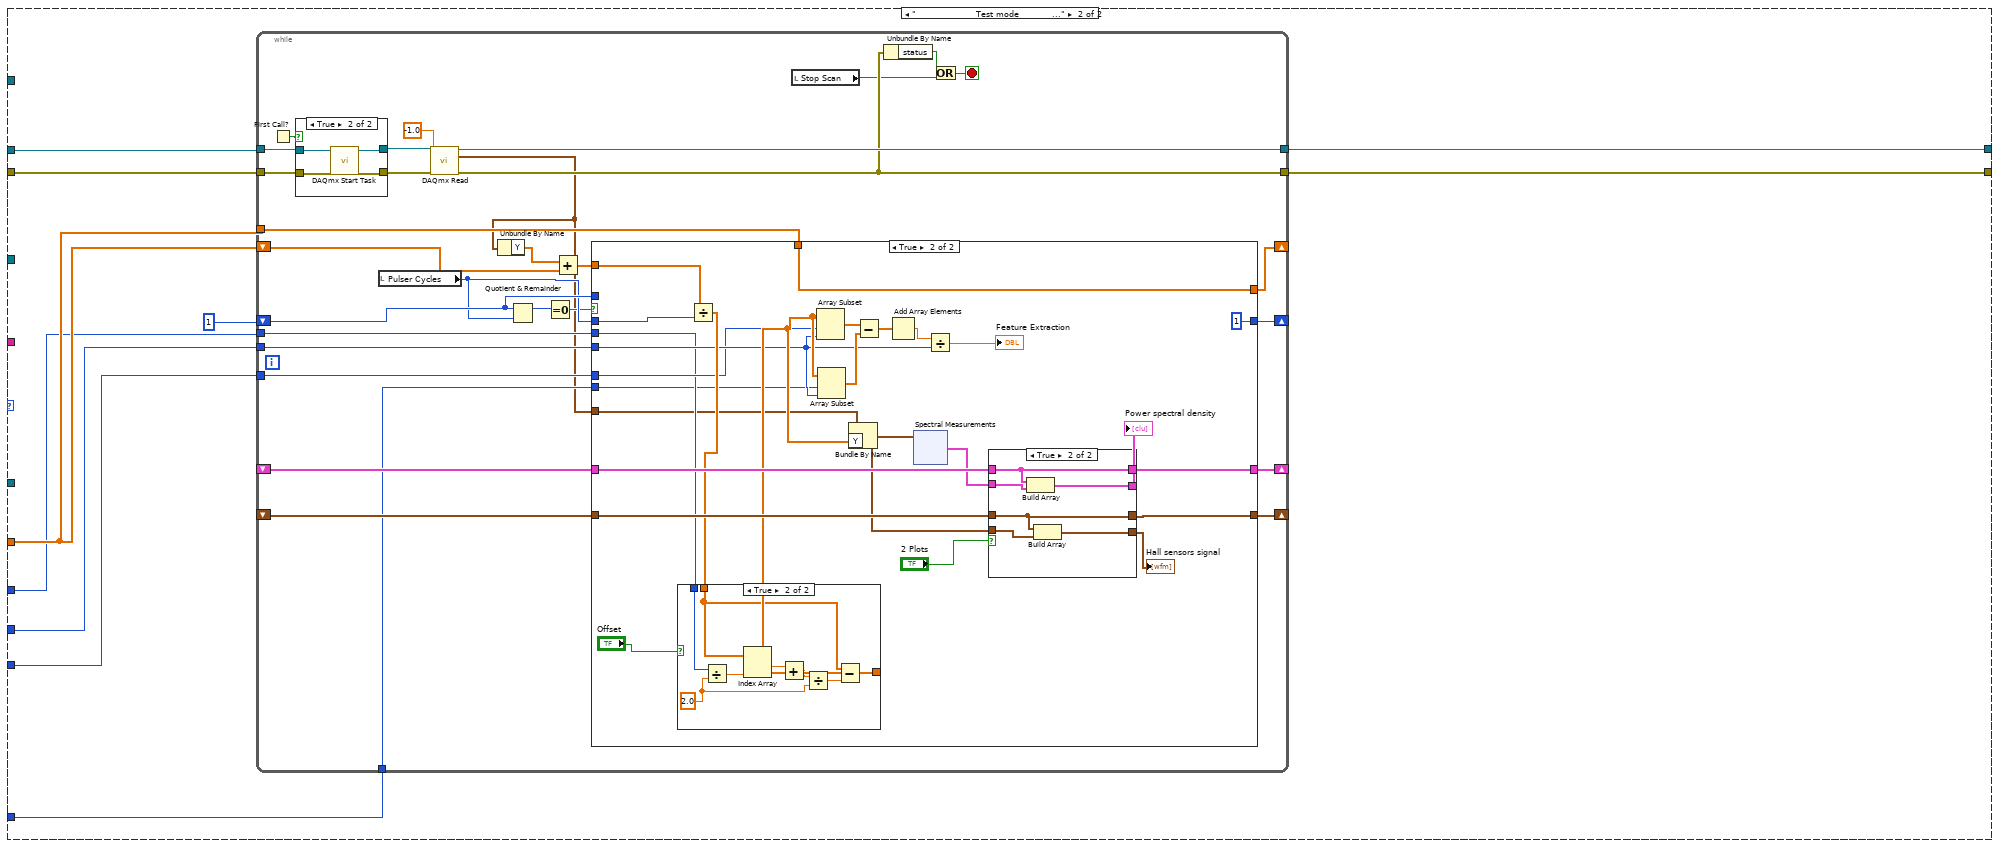
[diagram p20: hidden frame]
diagram:
  w69 = 10178 items=["Finite Samples"=10178, "Continuous Samples"=10123, "Hardware Timed Single Point"=12522]  # Sample Mode
  w83 = 15846 items=["Open"=10437, "Open or Create"=15846, "Create or Replace"=15847, "Create"=15848]  # Operation
  # "Counter pulses from Motor\nto pick up signal"
  # "1/2"
  # "start1"
  # "start2"
  # "Length"
  # "Mov. dis Y"
  # "Old. Pos Y"
  # "Mov. dis X"
  # "Old. Pos X"
  # "No. step = 5\n1p~0.004mm"
  # "Initial speed for 2 axes"
  # "Sigma Control"
  n1 = flat-sequence {
    tunnel: [w138] -> w46
    tunnel: [TRUE ("disable buffering (T)")] -> w3
    frame #0 {
      n2 = call "File Dialog"("prompt"="Choose New File For Recording\n" ("button label"), "default name"="PECT_default", "pattern (all files)"="*.tdms") -> ("selected path"=w120:path, "exists"=w115:bool, "cancelled"=w116:bool)  [unwired: 9 in, 1 out]
      n3 = case shown="False" w116 {
        tunnel: w120 -> [w121 _]
        tunnel: w115 -> [w122 _]
        frame False {
          n4 = case shown="True" w122 {
            tunnel: w121 -> [w123 w124]
            frame False {
              n5 = local write "Record path"(w123) -> ()
            }
            frame True {
              n6 = Two Button Dialog(message="Existing File\nDo you want to Replace?", 1:"No" ("F button name (\"Cancel\")"), 2:"Replace" ("T button name (\"OK\")")) -> (T button?=w125:bool)
              n7 = case shown="False" w125 {
                tunnel: w124 -> [_ w133]
                tunnel: [path "" ("deleted path") w132] -> w126
                frame False {
                  n8 = local write "Stop Scan"(TRUE ("Exit")) -> ()
                }
                frame True {
                  n9 = Delete(path (use dialog)=w133) -> (deleted path=w132:path)  [unwired: 4 in, 2 out]
                }
              }
              "Record path" <- w126
            }
          }
        }
        frame True {
          n10 = local write "Stop Scan"(TRUE ("Exit")) -> ()
        }
      }
    }
    frame #1 {
      n11 = local read "Record path"() -> (w137:path)
      n12 = local write "Completed"(FALSE ("Completed")) -> ()
      n13 = TDMS Open(6:FALSE ("disable buffering (T)"), 10:T5."create or replace" ("operation"), 11:w137) -> (3:w138:refnum<k34>)  [unwired: 3 in, 1 out]
    }
  }
  n14 = call-poly <vilib>:"DAQmx Create Virtual Channel.vi"("maximum value"="Max Voltage", "minimum value"="Min Voltage", "input terminal configuration"="Terminal Configuration", "physical channels"="Physical Channel") -> ("task out"=w86:refnum<k21>, "error out"=w87:errorcluster)  [unwired: 10 in]
  n15 = local read "Pulse generator"() -> (w30:T1)
  n16 = Unbundle By Name(w30) -> ("Frequency"=w50:dbl)
  n17 = local read "Pulse generator"() -> (w29:T1)
  n18 = Divide(x="Sample Rate", y=w50) -> (x/y=w49:dbl)
  n19 = Round Toward -Infinity(1:w49) -> (0:w41:dbl)
  "Sample per Channel AI" <- w41
  n20 = call-poly <vilib>:"DAQmx Timing.vi"("task/channels in"=w86, "sample mode"=w69, "samples per channel"=w41, "rate"="Sample Rate", "source"="Sample Clock Source 2", "error in"=w87) -> ("task out"=w1:refnum<k21>, "error out"=w88:errorcluster)  [unwired: 8 in]
  n21 = Unbundle By Name(w29) -> ("Frequency"=w42:dbl)
  n22 = property class="DAQmx Timing"(reference=w1, error in=w88) -> (reference out=w85:refnum<k21>, error out=w84:errorcluster, "SampClk.Rate"=w7:dbl)
  "Actual Sample Rate" <- w7
  n23 = call-poly <vilib>:"DAQmx Configure Logging.vi"("task/channels in"=w85, "operation"=w83, "file path"="TDMS File Path", "logging mode"="Logging Mode", "error in"=w84) -> ("task out"=w82:refnum<k21>, "error out"=w81:errorcluster)  [unwired: 9 in]
  n24 = call-poly "VISA Configure Serial Port"("VISA resource name"="COM Port", "baud rate (9600)"="Baud Rate", "data bits (8)"="Data bits", "parity (0:none)"="Parity", "stop bits (10: 1 bit)"="stop bits") -> ("VISA resource name out"=w101:refnum<visa-resource-name>, "error out"=w107:errorcluster)  [unwired: 9 in]
  n25 = local write "Direction (+)"(TRUE ("Scan")) -> ()
  n26 = local write "Scan"(FALSE ("Scan")) -> ()
  n27 = call-poly <vilib>:"DAQmx Trigger.vi"("task/channels in"=w82, "source"="Pulser Trigger Source", "edge"="Edge", "error in"=w81) -> ("task out"=w66:refnum<k21>, "error out"=w65:errorcluster)  [unwired: 10 in]
  n28 = call-poly <vilib>:"DAQmx Create Virtual Channel.vi"("counter"="Counter Pulse from Motor") -> ("task out"=w22:refnum<k21>, "error out"=w24:errorcluster)  [unwired: 13 in]
  n29 = VISA Set I/O Buffer Size(VISA resource name=w101, mask (16)=48, size (4096)=u32 8192, error in (no error)=w107) -> (VISA resource name out=w16:refnum<visa-resource-name>, error out=w15:errorcluster)
  n30 = property class="DAQmx Trigger"(reference=w66, error in=w65, "Start.Retriggerable"=TRUE) -> (reference out=w48:refnum<k21>, error out=w6:errorcluster)
  n31 = disable-structure shown="Disabled" {
    disable-tunnel: w6 -> [w149 _]
    frame Disabled {
      w170 = 10178 items=["Finite Samples"=10178, "Continuous Samples"=10123, "Hardware Timed Single Point"=12522]  # Sample Mode
      n32 = local read "Pulse generator"() -> (w143:T1)
      n33 = call-poly <vilib>:"DAQmx Create Virtual Channel.vi"("maximum value"="Max Voltage 2", "minimum value"="Min Voltage 2", "physical channels"="Physical Channel(s)", "error in"=w149) -> ("task out"=w159:refnum<k21>, "error out"=w158:errorcluster)  [unwired: 10 in]
      n34 = Unbundle By Name(w143) -> ("Frequency"=w155:dbl)
      n35 = Divide(x="Sample Rate 2", y=w155) -> (x/y=w153:dbl)
      n36 = Multiply(x="Pulser Cycles", y=w153) -> (x*y=w151:dbl)
      n37 = Round Toward -Infinity(1:w151) -> (0:w150:dbl)
      "Sample per Channel AO" <- w150
      n38 = call-poly <vilib>:"DAQmx Timing.vi"("task/channels in"=w159, "sample mode"=w170, "samples per channel"=w150, "rate"="Sample Rate 2", "source"="Sample Clock Source", "error in"=w158) -> ("task out"=w172:refnum<k21>, "error out"=w171:errorcluster)  [unwired: 8 in]
      n39 = property class="DAQmx Timing"(reference=w172, error in=w171) -> (reference out=w142:refnum<k21>, error out=w164:errorcluster, "SampClk.Rate"=w162:dbl)
      "Actual Sample Rate 2" <- w162
      n40 = Unbundle By Name("Pulse generator") -> ("Waveform Type"=w148:u16, "Frequency"=w147:dbl, "Amplitude"=w145:dbl)
      n41 = Bundle By Name(cluster=cluster{"Fs":dbl, "#s":dbl} {"Fs"=1000.0, "#s"=1000.0} ("sampling info"), "#s"=w150, "Fs"=w162) -> (w161:cluster{"Fs":dbl, "#s":dbl})
      n42 = call <vilib>:"Basic Function Generator.vi"("square wave duty cycle (%)"="Duty cycle %", "sampling info"=w161, "signal type"=w148, "error in (no error)"=w164, "amplitude"=w145, "frequency"=w147) -> ("error out"=w141:errorcluster, "signal out"=w160:waveform(dbl))  [unwired: 3 in, 1 out]
      "Waveform Graph 2" <- w160
      n43 = disable-structure shown="Enabled" {
        disable-tunnel: w160 -> [w177 w200]
        disable-tunnel: [w176 w199] -> w157
        disable-tunnel: [w175 w198] -> w156
        disable-tunnel: w142 -> [w174 w202]
        disable-tunnel: w141 -> [w173 w201]
        frame Disabled {
          n44 = while {
            tunnel: w177 -> [w188]
            shift-right: [w184] -> w176
            shift-left: w174 -> [w182]
            shift-right: [w183] -> w175
            shift-left: w173 -> [w181]
            stop <- FALSE stop-if-true
            n45 = call-poly <vilib>:"DAQmx Write.vi"("task/channels in"=w182, "data"=w188, "timeout"=-1.0, "error in"=w181) -> ("task out"=w187:refnum<k21>, "error out"=w186:errorcluster)  [unwired: 9 in, 1 out]
            n46 = call <vilib>:"DAQmx Start Task.vi"("task/channels in"=w187, "error in"=w186) -> ("task out"=w180:refnum<k21>, "error out"=w179:errorcluster)  [unwired: 12 in]
            n47 = disable-structure shown="Enabled" {
              disable-tunnel: [w194 w196] -> w184
              disable-tunnel: [w193 w195] -> w183
              disable-tunnel: w180 -> [w192 w196]
              disable-tunnel: w179 -> [w191 w195]
              frame Disabled {
                n48 = call <vilib>:"DAQmx Wait Until Done.vi"("task/channels in"=w192, "error in"=w191) -> ("task out"=w190:refnum<k21>, "error out"=w189:errorcluster)  [unwired: 12 in]
                n49 = call <vilib>:"DAQmx Stop Task.vi"("task/channels in"=w190, "error in"=w189) -> ("task out"=w194:refnum<k21>, "error out"=w193:errorcluster)  [unwired: 12 in]
              }
              frame Enabled {
              }
            }
          }
        }
        frame Enabled {
          n50 = call-poly <vilib>:"DAQmx Write.vi"("task/channels in"=w202, "data"=w200, "timeout"=-1.0, "error in"=w201) -> ("task out"=w204:refnum<k21>, "error out"=w206:errorcluster)  [unwired: 9 in, 1 out]
          n51 = call <vilib>:"DAQmx Start Task.vi"("task/channels in"=w204, "error in"=w206) -> ("task out"=w203:refnum<k21>, "error out"=w205:errorcluster)  [unwired: 12 in]
          n52 = while {
            tunnel: w203 -> [w214]
            tunnel: w205 -> [w213]
            tunnel: [w211] -> w198
            tunnel: [w212] -> w199
            stop <- w207 stop-if-true
            n53 = call <vilib>:"DAQmx Is Task Done.vi"("task/channels in"=w214, "error in"=w213) -> ("task out"=w212:refnum<k21>, "error out"=w211:errorcluster)  [unwired: 11 in, 1 out]
            n54 = Unbundle By Name(w211) -> ("status"=w208:bool)
            n55 = Wait Until Next ms Multiple(millisecond multiple=u32 100) -> ()  [unwired: 1 out]
            n56 = Compound Arithmetic op=OR(w208, "Stop 4") -> (w207:bool)
          }
        }
      }
      n57 = call <vilib>:"DAQmx Clear Task.vi"("task in"=w157, "error in"=w156) -> ("error out"=w169:errorcluster)  [unwired: 13 in]
      n58 = call <vilib>:"Simple Error Handler.vi"("error in (no error)"=w169) -> ()  [unwired: 4 in, 5 out]
    }
    frame Enabled {
    }
  }
  n59 = local read "Y-length"() -> (w53:dbl)
  n60 = local read "Step Y"() -> (w54:dbl)
  n61 = local read "X-length"() -> (w56:dbl)
  n62 = local read "Step X"() -> (w55:dbl)
  n63 = property class="DAQmx Channel"(reference=w22, error in=w24, "CI.CountEdges.Term"="Input Counter Terminal") -> (reference out=w17:refnum<k21>, error out=w18:errorcluster)
  n64 = call "Sigma_TriggerOff.vi"("error in (no error)"=w15, "VISA resource name"=w16) -> ("error out"=w13:errorcluster, "VISA resource name out"=w14:refnum<visa-resource-name>)  [unwired: 8 in]
  n65 = Quotient & Remainder(x=w53, y=w54) -> (floor(x/y)=w2:dbl)  [unwired: 1 out]
  n66 = Quotient & Remainder(x=w56, y=w55) -> (floor(x/y)=w44:dbl)  [unwired: 1 out]
  n67 = Build Array(w42, w7, w44, w2) -> (w12:dbl[])
  n68 = TDMS Write(0:w46, 5:"Freq_Sampling_SizeX_SizeY" ("group name in (Untitled)"), 9:w12) -> (4:w45:refnum<k34>)  [unwired: 3 in, 3 out]
  n69 = call "PECT_GateConverse.vi"("Gate 2"="Gate 2", "Gate 1"="Gate 1", "Freq_Sampling_SizeX_SizeY"=w12) -> ("Length T/2"=w31:i32, "Length"=w32:i32, "Start 2"=w33:i32, "Start 1"=w34:i32)  [unwired: 5 in]
  n70 = Obtain Queue(max queue size (-1, unlimited)=10000, name (unnamed)="data DAQ", element data type=dbl[] [] ("data")) -> (queue out=w61:refnum<queue>)  [unwired: 2 in, 2 out]
  n71 = Initialize Array(0.0 ("element"), w41) -> (w62:dbl[])
  n72 = Obtain Queue(name (unnamed)="data Extraction", element data type=0.0) -> (queue out=w59:refnum<queue>)  [unwired: 3 in, 2 out]
  n73 = Obtain Queue(max queue size (-1, unlimited)=2 ("최대 큐 크기(-1,제한없음)"), name (unnamed)="2D data", element data type=dbl[][] [] ("initialized array")) -> (queue out=w9:refnum<queue>)  [unwired: 2 in, 2 out]
  n74 = call "Sigma_SetSpeed.vi"("VISA resource name"=w14, "Travel per Pulse (0.004mm)"="Travel per Pulse (mm)", "Min (1mm) 2"="2 Min", "Max (2mm) 2"="2 Max", "Rate (1mm) 2"="2 Rate", "error in (no error)"=w13, "Axis (1)"="W", "Min (1mm)"="1 Min", "Max (2mm)"="1  Max", "Rate (1mm)"="1 Rate") -> ("VISA resource name out"=w113:refnum<visa-resource-name>, "error out"=w114:errorcluster)  [unwired: 8 in]
  n75 = case shown="\"                          Scan mode                      \", Default" "Tab Control 2" {
    tunnel: w48 -> [w249 w475]
    tunnel: [w248 w474] -> w72
    tunnel: [w247 w473] -> w71
    tunnel: w62 -> [w244 w472]
    tunnel: w6 -> [w246 w471]
    tunnel: w31 -> [w245 w470]
    tunnel: w61 -> [w243 _]
    tunnel: w59 -> [w222 _]
    tunnel: w44 -> [w217 _]
    tunnel: w2 -> [w218 _]
    tunnel: w32 -> [w230 w468]
    tunnel: w34 -> [w229 w467]
    tunnel: w33 -> [w228 w466]
    tunnel: w45 -> [w227 _]
    tunnel: "Waveform" ("group name in (Untitled)") -> [w224 _]
    tunnel: w9 -> [w219 _]
    frame "                          Scan mode                      ", Default {
      # "Column"
      # "Row"
      n76 = Initialize Array(0.0 ("element"), w217, w218) -> (w236:dbl[][])
      n77 = local read "3D Surface"() -> (w231:refnum<k7>)
      n78 = Matrix Size(0:w236) -> (1:w237:i32, 2:w238:i32)
      n79 = Decrement(x=w237) -> (x-1=w241:i32)
      n80 = Decrement(x=w238) -> (x-1=w240:i32)
      n81 = call "Surface_AxesScale.vi"("Y-axis Max"=w240, "X-axis max"=w241, "3D Surface"=w231, "Auto Scale"=FALSE) -> ()  [unwired: 8 in]
      n82 = while {
        shift-right: [w293] -> _
        shift-left: 0 -> [w295]
        shift-right: [w292] -> _
        shift-left: 0 -> [w294]
        tunnel: w222 -> [w291]
        shift-right: [w282] -> w215
        shift-left: w236 -> [w290]
        shift-right: [w285] -> _
        shift-left: TRUE ("Output Direction") -> [w286]
        tunnel: w219 -> [w284]
        tunnel: [w283] -> w220
        stop <- w288 stop-if-true
        n83 = local read "Scan"() -> (w281:bool)
        n84 = local read "Completed"() -> (w280:bool)
        n85 = Compound Arithmetic op=AND(invert w281, invert w280) -> (w279:bool)
        n86 = case shown="True" w279 {
          tunnel: w295 -> [w308 w343]
          tunnel: w294 -> [w307 w342]
          tunnel: [w306 w343] -> w293
          tunnel: [w300 w342] -> w292
          tunnel: w291 -> [w305 w334]
          tunnel: w290 -> [w304 w339]
          tunnel: [w297 w320] -> w282
          tunnel: [w303 _] -> w287
          tunnel: w286 -> [w302 w341]
          tunnel: [w301 w341] -> w285
          tunnel: w284 -> [w298 w322]
          tunnel: [w296 w334] -> w283
          frame False {
            n87 = Dequeue Element(queue=w305) -> (queue out=w296:refnum<queue>, element=w299:dbl)  [unwired: 2 in, 2 out]
            n88 = call "EletoMatr_1channel.vi"("Input Array X"=w304, "Input data"=w299, "In Row"=w308, "In Column"=w307, "Input Direction"=w302) -> ("Completed"=w303:bool, "Out Array X"=w297:dbl[][], "Out Row"=w306:i32, "Output Direction"=w301:bool, "Out Column"=w300:i32)  [unwired: 6 in]
            n89 = Lossy Enqueue Element(queue=w298, element=w297) -> ()  [unwired: 1 in, 4 out]
          }
          frame True {
            n90 = local read "Gate 1"() -> (w338:dbl)
            n91 = local read "Gate 2"() -> (w337:dbl)
            n92 = local read "Offset"() -> (w328:bool)
            n93 = Wait Until Next ms Multiple(millisecond multiple=u32 100 ("ms 배수")) -> ()  [unwired: 1 out]
            n94 = call "TDMS_Open.vi"("Offset"=w328, "Gate 2"=w337, "Gate 1"=w338, "Input 2D"=w339, "Open"="Open tdms") -> ("Output 2D"=w314:dbl[][])  [unwired: 5 in, 1 out]
            n95 = call "RepairLine.vi"("Repair Line Col"="Repair Line Col", "Repair Line Row"="Repair Line Row", "Line Col"="Line Col", "Line Row"="Line Row", "Array In"=w314) -> ("Array Repaired"=w313:dbl[][])  [unwired: 6 in]
            n96 = call "CSV Open.vi"("2D Array In"=w313, "Open"="Open csv") -> ("2D Array Out"=w321:dbl[][])  [unwired: 9 in]
            n97 = call "Backdata.vi"("Backindex"="Backindex", "Array in"=w321, "Backdata"="Backdata") -> ("Array out"=w325:dbl[][])
            n98 = call "Abs.vi"(10:"Inverse"=w325, 11:"Inverse"="Inverse") -> ("Array out"=w327:dbl[][])  [unwired: 9 in]
            n99 = call "DiffX.vi"("Array in"=w327, "DiffX"="DiffX") -> ("Array out"=w332:dbl[][])  [unwired: 1 in]
            n100 = call "DiffY.vi"("Array in"=w332, "DiffY"="DiffY") -> ("Array out"=w330:dbl[][])  [unwired: 1 in]
            n101 = call "Odd.vi"("Odd"="Odd", "Array In"=w330) -> ("Array Out"=w318:dbl[][])  [unwired: 9 in]
            n102 = call "Filter_Lowpass - 2D.vi"("Filter"="Filter", "Input 2D"=w318, "low cutoff freq: fl"="low cutoff freq: fl") -> ("Output"=w317:dbl[][])  [unwired: 6 in]
            n103 = case shown="True" TRUE {
              tunnel: w317 -> [w344 w345]
              tunnel: [w344 w345] -> w320
              tunnel: w322 -> [_ w346]
              frame False {
              }
              frame True {
                n104 = local read "3D Surface"() -> (w350:refnum<k7>)
                n105 = Matrix Size(0:w345) -> (1:w351:i32, 2:w348:i32)
                n106 = Decrement(x=w351) -> (x-1=w349:i32)
                n107 = Decrement(x=w348) -> (x-1=w347:i32)
                n108 = call "Surface_AxesScale.vi"("Y-axis Max"=w347, "X-axis max"=w349, "3D Surface"=w350, "Auto Scale"=FALSE) -> ()  [unwired: 8 in]
                n109 = Lossy Enqueue Element(queue=w346, element=w345) -> ()  [unwired: 1 in, 4 out]
              }
            }
          }
        }
        "Completed" <- w287
        n110 = local read "Stop Scan"() -> (w289:bool)
        n111 = Compound Arithmetic op=OR(w287, w289) -> (w288:bool)
        "No. Y" <- w294
        "No. X" <- w295
      }
      n112 = while {
        tunnel: w249 -> [w361]
        tunnel: [w360] -> w248
        tunnel: [w359] -> w247
        tunnel: w246 -> [w358]
        tunnel: w243 -> [w357]
        stop <- w353 stop-if-true
        n113 = case shown="True" "Scan" {
          tunnel: w361 -> [w363 w368]
          tunnel: [w363 w367] -> w360
          tunnel: [w362 w366] -> w359
          tunnel: w358 -> [w362 w365]
          tunnel: w357 -> [_ w364]
          frame False {
          }
          frame True {
            n114 = while {
              tunnel: w368 -> [w378]
              tunnel: [w381] -> w367
              tunnel: [w380] -> w366
              tunnel: w365 -> [w377]
              tunnel: w364 -> [w379]
              stop <- w369 stop-if-true
              n115 = First Call?() -> (First Call?: T/F=w374:bool)
              n116 = case shown="True" w374 {
                tunnel: w378 -> [w382 w387]
                tunnel: w377 -> [w383 w386]
                tunnel: [w382 w385] -> w376
                tunnel: [w383 w384] -> w375
                frame False {
                }
                frame True {
                  n117 = call <vilib>:"DAQmx Start Task.vi"("task/channels in"=w387, "error in"=w386) -> ("task out"=w385:refnum<k21>, "error out"=w384:errorcluster)  [unwired: 12 in]
                }
              }
              n118 = call-poly <vilib>:"DAQmx Read.vi"("task/channels in"=w376, "error in"=w375) -> ("task out"=w381:refnum<k21>, "data"=w373:dbl[], "error out"=w380:errorcluster)  [unwired: 11 in]
              n119 = Enqueue Element(queue=w379, element=w373) -> ()  [unwired: 2 in, 3 out]
              n120 = Unbundle By Name(w380) -> ("status"=w370:bool)
              n121 = local read "Completed"() -> (w372:bool)
              n122 = local read "Stop Scan"() -> (w371:bool)
              n123 = Compound Arithmetic op=OR(w370, w372, w371) -> (w369:bool)
            }
          }
        }
        n124 = local read "Completed"() -> (w354:bool)
        n125 = local read "Stop Scan"() -> (w355:bool)
        n126 = Compound Arithmetic op=OR(w354, w355) -> (w353:bool)
      }
      n127 = while {
        shift-right: [w404] -> _
        shift-left: w244 -> [w408]
        tunnel: w244 -> [w407]
        tunnel: w245 -> [w406]
        tunnel: w243 -> [w405]
        tunnel: w222 -> [w403]
        shift-right: [w400] -> _
        shift-left: 0 -> [w401]
        tunnel: w230 -> [w399]
        tunnel: w229 -> [w398]
        tunnel: w228 -> [w397]
        tunnel: w227 -> [w396]
        tunnel: [w395] -> w226
        tunnel: [w394] -> w225
        tunnel: w224 -> [w393]
        shift-right: [w391] -> _
        shift-left: 0 -> [w392]
        stop <- w388 stop-if-true
        n128 = local read "Scan"() -> (w402:bool)
        n129 = case shown="True" w402 {
          tunnel: w408 -> [w413 w426]
          tunnel: w407 -> [_ w432]
          tunnel: w406 -> [_ w431]
          tunnel: w405 -> [_ w430]
          tunnel: [w413 w429] -> w404
          tunnel: w403 -> [_ w428]
          tunnel: w401 -> [w412 w424]
          tunnel: [w412 w423] -> w400
          tunnel: w399 -> [_ w422]
          tunnel: w398 -> [_ w421]
          tunnel: w397 -> [_ w420]
          tunnel: w396 -> [w410 w419]
          tunnel: [w410 w418] -> w395
          tunnel: [_ w417] -> w394
          tunnel: w393 -> [_ w416]
          tunnel: w392 -> [w409 w415]
          tunnel: [w409 w414] -> w391
          frame False {
            n130 = Wait Until Next ms Multiple(millisecond multiple=u32 100 ("ms 배수")) -> ()  [unwired: 1 out]
          }
          frame True {
            n131 = local read "Pulser Cycles"() -> (w425:i32)
            n132 = Increment(x=w424) -> (x+1=w423:i32)
            n133 = Dequeue Element(queue=w430) -> (element=w427:dbl[])  [unwired: 2 in, 3 out]
            n134 = Quotient & Remainder(x=w423, y=w425) -> (x-y*floor(x/y)=w433:i32)  [unwired: 1 out]
            n135 = Add(x=w427, y=w426) -> (x+y=w435:dbl[])
            n136 = Equal To 0?(x=w433) -> (x = 0?=w434:bool)
            n137 = case shown="True" w434 {
              tunnel: w425 -> [_ w456]
              tunnel: w435 -> [w438 w454]
              tunnel: [w438 w457] -> w429
              tunnel: w432 -> [_ w457]
              tunnel: w431 -> [_ w450]
              tunnel: w428 -> [_ w455]
              tunnel: w422 -> [_ w451]
              tunnel: w421 -> [_ w453]
              tunnel: w420 -> [_ w452]
              tunnel: w419 -> [w437 w444]
              tunnel: [w437 w441] -> w418
              tunnel: [_ w440] -> w417
              tunnel: w416 -> [_ w443]
              tunnel: w415 -> [w436 w446]
              tunnel: [w436 w445] -> w414
              frame False {
                n138 = disable-structure shown="비활성화" {
                  frame Disabled {
                    n139 = Wait Until Next ms Multiple(millisecond multiple=u32 100 ("ms 배수")) -> ()  [unwired: 1 out]
                  }
                  frame Enabled {
                  }
                }
              }
              frame True {
                n140 = Divide(x=w454, y=w456) -> (x/y=w442:dbl[])
                n141 = local read "Offset"() -> (w449:bool)
                n142 = local read "Motor Pulse Count"() -> (w445:i32)
                n143 = call "PECT_Feature extraction.vi"("Length T/2"=w450, "Offset"=w449, "Length"=w451, "Start 2"=w452, "Start 1"=w453, "Pulse signal in"=w442) -> ("Feature extraction out"=w448:dbl)  [unwired: 5 in]
                n144 = Not Equal?(x=w445, y=w446) -> (x != y?=w447:bool)
                n145 = case shown="True" w447 {
                  tunnel: w455 -> [_ w465]
                  tunnel: w448 -> [_ w464]
                  tunnel: w444 -> [w458 w463]
                  tunnel: w443 -> [_ w462]
                  tunnel: w442 -> [_ w461]
                  tunnel: [w458 w460] -> w441
                  tunnel: [_ w459] -> w440
                  frame False {
                  }
                  frame True {
                    n146 = TDMS Write(0:w463, 5:w462, 9:w461) -> (4:w460:refnum<k34>, 15:w459:errorcluster)  [unwired: 3 in, 2 out]
                    n147 = Enqueue Element(queue=w465, element=w464) -> ()  [unwired: 2 in, 3 out]
                  }
                }
              }
            }
          }
        }
        n148 = local read "Completed"() -> (w390:bool)
        n149 = local read "Stop Scan"() -> (w389:bool)
        n150 = Compound Arithmetic op=OR(w390, w389) -> (w388:bool)
        "No.data" <- w401
      }
      n151 = while {
        tunnel: w219 -> [w271]
        tunnel: w218 -> [_]
        tunnel: w217 -> [_]
        tunnel: [w268] -> w216
        stop <- w269 stop-if-true
        n152 = local read "No. Y"() -> (w273:i32)
        n153 = Dequeue Element(queue=w271) -> (queue out=w268:refnum<queue>, element=w267:dbl[][])  [unwired: 2 in, 2 out]
        n154 = Index Array(array=w267, index (col)=w273) -> (element=→"Feature extraction scan":dbl[])  [unwired: 1 in]
        n155 = call <vilib>:"3D Surface.vi"("z matrix"=w267, "3D graph"="3D Surface") -> ()  [unwired: 8 in, 2 out]
        n156 = local read "Completed"() -> (w266:bool)
        n157 = case shown="True" w266 {
          selector: w266 -> [w276 w277]
          tunnel: [w276 w277] -> w265
          frame False {
          }
          frame True {
            n158 = Wait (ms)(milliseconds to wait=u32 200) -> ()  [unwired: 1 out]
          }
        }
        n159 = local read "Stop Scan"() -> (w270:bool)
        n160 = Compound Arithmetic op=OR(w265, w270) -> (w269:bool)
        n161 = Wait Until Next ms Multiple(millisecond multiple=u32 100 ("ms 배수")) -> ()  [unwired: 1 out]
      }
      n162 = Release Queue(queue=w216) -> ()  [unwired: 2 in, 3 out]
      n163 = while {
        stop <- w254 stop-if-true
        n164 = event shown="[2] \"Max\", \"Min\", \"ColorMapAutoScale\": Value Change" {
          selector: _ -> [_ _ _]
          dyn-events: _ -> [_ _ _]
          timeout: _ -> [_ _ _]
          tunnel: [_ w258 _] -> w254
          event "Plot style", "ViewMode": Value Change {
            n165 = event-data() -> ()  [unwired: 1 in, 2 out]
            n166 = local read "3D Surface"() -> (w257:refnum<k7>)
            n167 = property class="CWGraph3D"(reference=w257, "ViewMode"="ViewMode") -> ()  [unwired: 1 in, 2 out]
            n168 = call <vilib>:"Basic Properties.vi"("3D graph"=w257, "plot style"="Plot style") -> ()  [unwired: 12 in, 2 out]
          }
          event "Stop Scan": Value Change {
            n169 = event-data() -> ()  [unwired: 1 in, 5 out]
            n170 = local read "Stop Scan"() -> (w258:bool)
          }
          event "Max", "Min", "ColorMapAutoScale": Value Change {
            n171 = event-data() -> ()  [unwired: 1 in, 5 out]
            n172 = local read "3D Surface"() -> (w259:refnum<k7>)
            n173 = call "Surface_ColorScale.vi"("ColorMapAutoScale"="ColorMapAutoScale", "Min"="Min", "Max"="Max", "3D Surface_"=w259) -> ("Min 2"=w263:dbl, "Max 2"=w262:dbl)  [unwired: 1 in, 2 out]
            n174 = local write "Max"(w262) -> ()
            n175 = local write "Min"(w263) -> ()
          }
        }
      }
      n176 = TDMS Close(8:w225, 11:w226) -> (0:w223:errorcluster)  [unwired: 1 out]
      n177 = disable-structure shown="Disabled" {
        frame Disabled {
          n178 = global read "Global_data.vi" "global 2d graph"() -> ()  [unwired: 1 in]
        }
        frame Enabled {
        }
      }
      n179 = call <vilib>:"Simple Error Handler.vi"("error in (no error)"=w223) -> ()  [unwired: 2 in, 7 out]
      n180 = Release Queue(queue=w220) -> ()  [unwired: 2 in, 3 out]
      n181 = while {
        tunnel: w215 -> [w252]
        stop <- w251 stop-if-true
        n182 = call "CSV Save.vi"("Array"=w252, "Save Button"="Save Scan mode") -> ()  [unwired: 9 in, 1 out]
        n183 = Wait Until Next ms Multiple(millisecond multiple=u32 100 ("ms 배수")) -> ()  [unwired: 1 out]
        n184 = local read "Stop Scan"() -> (w251:bool)
      }
    }
    frame "                    Test mode                   " {
      n185 = while {
        tunnel: w475 -> [w485]
        tunnel: w471 -> [w484]
        tunnel: [w503] -> w473
        tunnel: [w504] -> w474
        shift-right: [w499] -> _
        shift-left: w472 -> [w500]
        tunnel: w472 -> [w498]
        shift-right: [w496] -> _
        shift-left: _ -> [w495]
        tunnel: w470 -> [w494]
        shift-right: [w493] -> _
        shift-left: _ -> [w492]
        shift-right: [w489] -> _
        shift-left: 1 ("Average") -> [w488]
        tunnel: w468 -> [w481]
        tunnel: w467 -> [w480]
        tunnel: w466 -> [w479]
        stop <- w505 stop-if-true
        n186 = First Call?() -> (First Call?: T/F=w486:bool)
        n187 = case shown="True" w486 {
          tunnel: w485 -> [w506 w511]
          tunnel: w484 -> [w507 w510]
          tunnel: [w506 w509] -> w483
          tunnel: [w507 w508] -> w482
          frame False {
          }
          frame True {
            n188 = call <vilib>:"DAQmx Start Task.vi"("task/channels in"=w511, "error in"=w510) -> ("task out"=w509:refnum<k21>, "error out"=w508:errorcluster)  [unwired: 12 in]
          }
        }
        n189 = local read "Pulser Cycles"() -> (w487:i32)
        n190 = call-poly <vilib>:"DAQmx Read.vi"("task/channels in"=w483, "timeout"=-1.0, "error in"=w482) -> ("task out"=w504:refnum<k21>, "data"=w477:waveform(dbl), "error out"=w503:errorcluster)  [unwired: 10 in]
        n191 = Unbundle By Name(w477) -> ("Y"=w476:dbl[])
        n192 = Quotient & Remainder(x=w488, y=w487) -> (x-y*floor(x/y)=w501:i32)  [unwired: 1 out]
        n193 = Equal To 0?(x=w501) -> (x = 0?=w478:bool)
        n194 = Add(x=w476, y=w500) -> (x+y=w497:dbl[])
        n195 = case shown="True" w478 {
          tunnel: w487 -> [_ w528]
          tunnel: w477 -> [_ w517]
          tunnel: w497 -> [w516 w542]
          tunnel: [w516 w541] -> w499
          tunnel: w498 -> [_ w541]
          tunnel: [w515 w539] -> w496
          tunnel: w495 -> [w515 w540]
          tunnel: w494 -> [_ w524]
          tunnel: [w514 w536] -> w493
          tunnel: w492 -> [w514 w537]
          tunnel: [w512 1 ("Average")] -> w489
          tunnel: w488 -> [w513 _]
          tunnel: w481 -> [_ w526]
          tunnel: w480 -> [_ w525]
          tunnel: w479 -> [_ w523]
          frame False {
            n196 = Increment(x=w513) -> (x+1=w512:i32)
          }
          frame True {
            n197 = Divide(x=w542, y=w528) -> (x/y=w531:dbl[])
            n198 = case shown="True" "Offset" {
              tunnel: w524 -> [_ w570]
              tunnel: w531 -> [w562 w564]
              tunnel: [w562 w563] -> w529
              frame False {
              }
              frame True {
                w566 = 2.0 ("y")
                n199 = Divide(x=w570, y=w566) -> (x/y=w571:dbl)
                n200 = Index Array(array=w564, index #2=w571) -> (element #1=w568:dbl, element #2=w569:dbl)  [unwired: 1 in]
                n201 = Add(x=w568, y=w569) -> (x+y=w567:dbl)
                n202 = Divide(x=w567, y=w566) -> (x/y=w565:dbl)
                n203 = Subtract(x=w564, y=w565) -> (x-y=w563:dbl[])
              }
            }
            n204 = Array Subset(array=w529, index=w525, length=w526) -> (w535:dbl[])
            n205 = Array Subset(array=w529, index=w523, length=w526) -> (w534:dbl[])
            n206 = Bundle By Name(cluster=w517, "Y"=w529) -> (w518:waveform(dbl))
            n207 = Subtract(x=w535, y=w534) -> (x-y=w533:dbl[])
            n208 = Add Array Elements(numeric array=w533) -> (sum=w538:dbl)
            n209 = xnode "Spectral Measurements"("신호"=w518) -> ("PSD"=w520:cluster{"f0":dbl, "df":dbl, "magnitude":dbl[]})  [unwired: 1 in, 1 out]
            n210 = Divide(x=w538, y=w526) -> (x/y=→"Feature Extraction":dbl)
            n211 = case shown="True" "2 Plots" {
              tunnel: [w546 w552] -> w522
              tunnel: w540 -> [_ w551]
              tunnel: [w545 w551] -> w539
              tunnel: w518 -> [w545 w547]
              tunnel: w520 -> [w543 w549]
              tunnel: [w544 w550] -> w519
              tunnel: w537 -> [_ w548]
              tunnel: [w543 w548] -> w536
              frame False {
                n212 = Build Array(w543, w543) -> (w544:cluster{"f0":dbl, "df":dbl, "magnitude":dbl[]}[])
                n213 = Build Array(w545, w545) -> (w546:waveform(dbl)[])
              }
              frame True {
                n214 = Build Array(w548, w549) -> (w550:cluster{"f0":dbl, "df":dbl, "magnitude":dbl[]}[])
                n215 = Build Array(w551, w547) -> (w552:waveform(dbl)[])
              }
            }
            "Power spectral density" <- w519
            "Hall sensors signal" <- w522
          }
        }
        n216 = local read "Stop Scan"() -> (w491:bool)
        n217 = Unbundle By Name(w503) -> ("status"=w502:bool)
        n218 = Or(x=w502, y=w491) -> (x .or. y?=w505:bool)
      }
    }
  }
  n219 = call <vilib>:"DAQmx Start Task.vi"("task/channels in"=w17, "error in"=w18) -> ("task out"=w19:refnum<k21>, "error out"=w5:errorcluster)  [unwired: 12 in]
  n220 = while {
    tunnel: w19 -> [w582]
    tunnel: w5 -> [w581]
    tunnel: [w573] -> w26
    tunnel: [w580] -> w25
    tunnel: [w572] -> _
    tunnel: w3 -> [w572]
    stop <- w574 stop-if-true
    n221 = call-poly <vilib>:"DAQmx Read.vi"("task/channels in"=w582, "error in"=w581) -> ("task out"=w580:refnum<k21>, "data"=→"Motor Pulse Count":u32, "error out"=w573:errorcluster)  [unwired: 11 in]
    n222 = Wait Until Next ms Multiple(millisecond multiple=u32 10 ("milliseconds to wait")) -> ()  [unwired: 1 out]
    n223 = local read "Completed"() -> (w575:bool)
    n224 = Unbundle By Name(w573) -> ("status"=w577:bool)
    n225 = local read "Stop Scan"() -> (w576:bool)
    n226 = Compound Arithmetic op=OR(w577, w575, w576) -> (w574:bool)
  }
  n227 = while {
    shift-right: [w599] -> _
    shift-left: T2."No Scan" -> [w600]
    shift-right: [w595] -> _
    shift-left: 0.0 ("Current  Position (mm)") -> [w594]
    shift-right: [w593] -> _
    shift-left: 0.0 ("Current  Position (mm)") -> [w592]
    shift-right: [w591] -> _
    shift-left: 0.0 ("Current  Position (mm)") -> [w590]
    shift-right: [w589] -> _
    shift-left: 0.0 ("Current  Position (mm)") -> [w588]
    shift-right: [w596] -> w38
    shift-left: w113 -> [w598]
    shift-right: [w585] -> w39
    shift-left: w114 -> [w597]
    tunnel: w3 -> [_]
    i -> [w587]
    stop <- w583 stop-if-true
    n228 = case shown="\"Wait to destinatioin Y\"" w600 {
      selector: w600 -> [w611 _ _ _ _]
      tunnel: [w612 T2."Wait to destination X" w676 T2."Wait to destinatioin Y" w727] -> w599
      tunnel: w598 -> [w606 w645 w670 w705 w718]
      tunnel: w597 -> [w605 w644 w669 w704 w717]
      tunnel: [w608 w647 w675 w695 w724] -> w596
      tunnel: [w607 w646 w674 w694 w723] -> w585
      tunnel: [w604 w652 w673 w701 w730] -> w595
      tunnel: w594 -> [w602 w652 w661 w701 w730]
      tunnel: [w610 w651 w678 w700 w729] -> w593
      tunnel: w592 -> [w601 w651 w678 w700 w729]
      tunnel: [w603 w650 w671 w699 w726] -> w591
      tunnel: w590 -> [_ w650 w671 w699 w712]
      tunnel: [w609 w649 w679 w698 w725] -> w589
      tunnel: w588 -> [_ w649 w679 w698 w725]
      frame "No Scan", Default {
        n229 = local read "Scan"() -> (w613:bool)
        n230 = case shown="True" w613 {
          tunnel: [w619 T2."Move X"] -> w612
          tunnel: w611 -> [w619 _]
          tunnel: w606 -> [w618 w625]
          tunnel: w605 -> [w617 w624]
          tunnel: [w618 w630] -> w608
          tunnel: [w617 w629] -> w607
          tunnel: [w616 w621] -> w604
          tunnel: [w615 w620] -> w603
          tunnel: w602 -> [w616 _]
          tunnel: w601 -> [w615 _]
          frame False {
            n231 = Wait (ms)(milliseconds to wait=u32 100) -> ()  [unwired: 1 out]
          }
          frame True {
            n232 = local read "Cur. Pos X"() -> (w627:dbl)
            n233 = local read "Cur. Pos Y"() -> (w628:dbl)
            n234 = local read "Travel per Pulse (mm)"() -> (w626:dbl)
            n235 = call "Sigma_GetPos.vi"("VISA resource name"=w625, "Travel per Pulse (mm)"=w626, "Init Pos X (mm)"=w627, "Init  Pos Y (mm)"=w628, "error in (no error)"=w624) -> ("Pos X (mm)"=w621:dbl, "Pos Y (mm)"=w620:dbl, "VISA resource name out"=w623:refnum<visa-resource-name>, "error out"=w622:errorcluster)  [unwired: 6 in, 1 out]
            "Start Pos. X" <- w621
            "Start. Pos.Y" <- w620
            n236 = local write "Cur. Pos X"(w621) -> ()
            n237 = local write "Cur. Pos Y"(w620) -> ()
            n238 = local read "Travel per Pulse (mm)"() -> (w633:dbl)
            n239 = local read "Step X"() -> (w634:dbl)
            n240 = local write "Direction (+)"(TRUE ("Direction (+)")) -> ()
            n241 = local write "Move X"(TRUE ("Move X")) -> ()
            n242 = call "Sigma_TriggerOut.vi"("Axis(1)"=1, "error in (no error)"=w622, "Trigger distance (mm)"=w634, "Travel per Pulse (mm)"=w633, "VISA resource name"=w623) -> ("error out"=w631:errorcluster, "VISA resource name out"=w632:refnum<visa-resource-name>)  [unwired: 5 in]
            n243 = flat-sequence {
              tunnel: [w641] -> w630
              tunnel: w632 -> [w641]
              tunnel: [w640] -> w629
              tunnel: w631 -> [w640]
              frame #0 {
                n244 = Wait (ms)(milliseconds to wait=u32 100) -> ()  [unwired: 1 out]
              }
            }
          }
        }
        n245 = local read "X-length"() -> (w610:dbl)
        n246 = local read "Step Y"() -> (w609:dbl)
      }
      frame "Move X" {
        n247 = local read "Travel per Pulse (mm)"() -> (w654:dbl)
        n248 = local read "X-length"() -> (w655:dbl)
        n249 = call "Sigma_MoveAbs.vi"("Direction (+)"="Direction (+)", "Axis (1)"=1, "error in (no error)"=w644, "Travel (1mm)"=w655, "Travel per Pulse (0.004mm)"=w654, "VISA resource name"=w645) -> ("error out"=w642:errorcluster, "VISA resource name out"=w643:refnum<visa-resource-name>)  [unwired: 4 in]
        n250 = flat-sequence {
          tunnel: [w659] -> w647
          tunnel: w643 -> [w659]
          tunnel: [w658] -> w646
          tunnel: w642 -> [w658]
          frame #0 {
            n251 = Wait (ms)(milliseconds to wait=u32 100) -> ()  [unwired: 1 out]
          }
        }
      }
      frame "Wait to destination X" {
        n252 = local read "Cur. Pos X"() -> (w666:dbl)
        n253 = local read "Cur. Pos Y"() -> (w665:dbl)
        n254 = local read "Travel per Pulse (mm)"() -> (w672:dbl)
        n255 = call "Sigma_GetPos.vi"("VISA resource name"=w670, "Travel per Pulse (mm)"=w672, "Init Pos X (mm)"=w666, "Init  Pos Y (mm)"=w665, "error in (no error)"=w669) -> ("Pos X (mm)"=w660:dbl, "Pos Y (mm)"=w664:dbl, "VISA resource name out"=w668:refnum<visa-resource-name>, "error out"=w667:errorcluster)  [unwired: 6 in, 1 out]
        "Cur. X" <- w660
        n256 = Absolute Value(x=w678) -> (abs(x)=w680:dbl)
        "move X" <- w680
        n257 = local write "Cur. Pos X"(w660) -> ()
        n258 = local write "Cur. Pos Y"(w664) -> ()
        n259 = Subtract(x=w660, y=w661) -> (x-y=w682:dbl)
        n260 = Absolute Value(x=w682) -> (abs(x)=w681:dbl)
        "delta X" <- w681
        n261 = Subtract(x=w681, y=w680) -> (x-y=w663:dbl)
        n262 = call "Convert Double Precision.vi"("Input"=w663) -> ("Output"=w662:dbl)  [unwired: 10 in]
        "Compare X" <- w662
        n263 = Greater Or Equal To 0?(x=w662) -> (x >= 0?=w677:bool)
        "x >= 0" <- w677
        n264 = case shown="False" w677 {
          tunnel: [T2."Wait to destination X" T2."Move Y"] -> w676
          tunnel: w668 -> [w685 w689]
          tunnel: w667 -> [w684 w688]
          tunnel: [w685 w689] -> w675
          tunnel: [w684 w688] -> w674
          tunnel: [w683 w690] -> w673
          tunnel: w661 -> [w683 _]
          frame False {
            n265 = disable-structure shown="비활성화" {
              frame Disabled {
                n266 = Wait (ms)(milliseconds to wait=u32 100) -> ()  [unwired: 1 out]
              }
              frame Enabled {
              }
            }
          }
          frame True {
            n267 = local read "Cur. Pos X"() -> (w690:dbl)
            n268 = local write "Move X"(FALSE ("Move X")) -> ()
          }
        }
        "Old X" <- w661
      }
      frame "Move Y" {
        n269 = local read "Travel per Pulse (mm)"() -> (w703:dbl)
        n270 = local read "Step Y"() -> (w706:dbl)
        n271 = call "Sigma_MoveAbs.vi"("Direction (+)"=TRUE, "Axis (1)"=2, "error in (no error)"=w704, "Travel (1mm)"=w706, "Travel per Pulse (0.004mm)"=w703, "VISA resource name"=w705) -> ("error out"=w696:errorcluster, "VISA resource name out"=w697:refnum<visa-resource-name>)  [unwired: 4 in]
        n272 = flat-sequence {
          tunnel: [w710] -> w695
          tunnel: w697 -> [w710]
          tunnel: [w709] -> w694
          tunnel: w696 -> [w709]
          frame #0 {
            n273 = Wait (ms)(milliseconds to wait=u32 100) -> ()  [unwired: 1 out]
          }
        }
      }
      frame "Wait to destinatioin Y" {
        n274 = local read "Cur. Pos X"() -> (w721:dbl)
        n275 = local read "Cur. Pos Y"() -> (w720:dbl)
        n276 = local read "Travel per Pulse (mm)"() -> (w722:dbl)
        n277 = call "Sigma_GetPos.vi"("VISA resource name"=w718, "Travel per Pulse (mm)"=w722, "Init Pos X (mm)"=w721, "Init  Pos Y (mm)"=w720, "error in (no error)"=w717) -> ("Pos X (mm)"=w719:dbl, "Pos Y (mm)"=w711:dbl, "VISA resource name out"=w716:refnum<visa-resource-name>, "error out"=w715:errorcluster)  [unwired: 6 in, 1 out]
        "Cur. Y" <- w711
        n278 = Absolute Value(x=w725) -> (abs(x)=w731:dbl)
        "move Y" <- w731
        n279 = Subtract(x=w711, y=w712) -> (x-y=w733:dbl)
        n280 = local write "Cur. Pos X"(w719) -> ()
        n281 = local write "Cur. Pos Y"(w711) -> ()
        n282 = Absolute Value(x=w733) -> (abs(x)=w732:dbl)
        "deltaY" <- w732
        n283 = Subtract(x=w732, y=w731) -> (x-y=w714:dbl)
        n284 = call "Convert Double Precision.vi"("Input"=w714) -> ("Output"=w713:dbl)  [unwired: 10 in]
        "compareY" <- w713
        n285 = Greater Or Equal To 0?(x=w713) -> (x >= 0?=w728:bool)
        "y >= 0" <- w728
        n286 = case shown="True" w728 {
          tunnel: [T2."Wait to destinatioin Y" w756] -> w727
          tunnel: w712 -> [w736 w752]
          tunnel: [w736 w749] -> w726
          tunnel: [w735 w747] -> w724
          tunnel: [w734 w746] -> w723
          tunnel: w716 -> [w735 w745]
          tunnel: w715 -> [w734 w744]
          frame False {
            n287 = disable-structure shown="비활성화" {
              frame Disabled {
                n288 = Wait (ms)(milliseconds to wait=u32 100) -> ()  [unwired: 1 out]
              }
              frame Enabled {
              }
            }
          }
          frame True {
            n289 = local read "Y-length"() -> (w741:dbl)
            n290 = local read "Step Y"() -> (w739:dbl)
            n291 = local read "Cur. Pos Y"() -> (w749:dbl)
            n292 = local read "Start. Pos.Y"() -> (w748:dbl)
            n293 = Subtract(x=w741, y=w739) -> (x-y=w740:dbl)
            n294 = Subtract(x=w748, y=w752) -> (x-y=w755:dbl)
            n295 = Absolute Value(x=w740) -> (abs(x)=w753:dbl)
            n296 = Absolute Value(x=w755) -> (abs(x)=w754:dbl)
            n297 = Subtract(x=w754, y=w753) -> (x-y=w742:dbl)
            n298 = local write "Move X"(FALSE ("Move X")) -> ()
            n299 = call "Convert Double Precision.vi"("Input"=w742) -> ("Output"=w743:dbl)  [unwired: 10 in]
            n300 = Greater Or Equal To 0?(x=w743) -> (x >= 0?=w750:bool)
            n301 = case shown="True" w750 {
              tunnel: [T2."Move X" T2."No Scan"] -> w756
              tunnel: [w758 w765] -> w747
              tunnel: [w757 w764] -> w746
              tunnel: w745 -> [w758 w763]
              tunnel: w744 -> [w757 w762]
              frame False {
                n302 = local read "Direction (+)"() -> (w760:bool)
                n303 = Not(x=w760) -> (.not. x?=w759:bool)
                n304 = local write "Direction (+)"(w759) -> ()
              }
              frame True {
                n305 = call "Sigma_TriggerOff.vi"("error in (no error)"=w762, "VISA resource name"=w763) -> ("error out"=w764:errorcluster, "VISA resource name out"=w765:refnum<visa-resource-name>)  [unwired: 8 in]
                n306 = local write "Scan"(FALSE ("Move X")) -> ()
              }
            }
          }
        }
        "Old.Y" <- w712
      }
    }
    n307 = Unbundle By Name(w585) -> ("status"=w584:bool)
    n308 = local read "Stop Scan"() -> (w586:bool)
    n309 = Compound Arithmetic op=OR(w584, w586) -> (w583:bool)
    "열거형" <- w600
    "숫자형" <- w587
  }
  n310 = while {
    shift-right: [w770] -> _
    shift-left: w113 -> [w775]
    shift-right: [w772] -> _
    shift-left: w114 -> [w774]
    stop <- w771 stop-if-true
    n311 = event shown="[1] \"Stop Scan\": Value Change" {
      selector: _ -> [_ _ _ _ _ _ _ _ _ _ _]
      dyn-events: _ -> [_ _ _ _ _ _ _ _ _ _ _]
      timeout: 100 -> [_ _ _ _ _ _ _ _ _ _ _]
      tunnel: w775 -> [w780 w813 w826 w829 w844 w859 w874 w891 w903 w913 w925]
      tunnel: w774 -> [w779 w812 w823 w828 w843 w858 w873 w890 w902 w912 w924]
      tunnel: [w778 w813 w825 w831 w846 w861 w876 w888 w901 w915 w927] -> w770
      tunnel: [w777 w812 w824 w830 w845 w860 w875 w887 w900 w914 w926] -> w772
      tunnel: [_ "Stop Scan" _ _ _ _ _ _ _ _ _] -> w769
      event Timeout {
        n312 = event-data() -> ()  [unwired: 1 in, 2 out]
        n313 = local read "Scan"() -> (w776:bool)
        n314 = case shown="False" w776 {
          tunnel: w780 -> [w792 w811]
          tunnel: w779 -> [w791 w810]
          tunnel: [w790 w811] -> w778
          tunnel: [w789 w810] -> w777
          frame False {
            # "Stop at LS"
            n315 = local read "Travel per Pulse (mm)"() -> (w784:dbl)
            n316 = local read "Cur. Pos X"() -> (w782:dbl)
            n317 = local read "Cur. Pos Y"() -> (w781:dbl)
            n318 = call "Sigma_GetPos.vi"("VISA resource name"=w792, "Travel per Pulse (mm)"=w784, "Init Pos X (mm)"=w782, "Init  Pos Y (mm)"=w781, "error in (no error)"=w791) -> ("Pos X (mm)"=w787:dbl, "Pos Y (mm)"=w788:dbl, "VISA resource name out"=w785:refnum<visa-resource-name>, "State String"=w783:string, "error out"=w786:errorcluster)  [unwired: 6 in]
            n319 = local write "Cur. Pos X"(w787) -> ()
            n320 = local write "Cur. Pos Y"(w788) -> ()
            n321 = case shown="\"W\"" w783 {
              tunnel: [w794 w799 w804 w809] -> w790
              tunnel: [w793 w798 w803 w808] -> w789
              tunnel: w785 -> [w794 w796 w801 w806]
              tunnel: w786 -> [w793 w795 w800 w805]
              frame "K", Default {
              }
              frame "L" {
                n322 = call "Sigma_Stop.vi"("Axis (1)"="1", "error in (no error)"=w795, "VISA resource name"=w796) -> ("error out"=w798:errorcluster, "VISA resource name out"=w799:refnum<visa-resource-name>)  [unwired: 7 in]
              }
              frame "M" {
                n323 = call "Sigma_Stop.vi"("Axis (1)"="2", "error in (no error)"=w800, "VISA resource name"=w801) -> ("error out"=w803:errorcluster, "VISA resource name out"=w804:refnum<visa-resource-name>)  [unwired: 7 in]
              }
              frame "W" {
                n324 = call "Sigma_Stop.vi"("Axis (1)"="W", "error in (no error)"=w805, "VISA resource name"=w806) -> ("error out"=w808:errorcluster, "VISA resource name out"=w809:refnum<visa-resource-name>)  [unwired: 7 in]
              }
            }
          }
          frame True {
          }
        }
      }
      event "Stop Scan": Value Change {
        n325 = event-data() -> ()  [unwired: 1 in, 2 out]
      }
      event "Save Speed": Value Change {
        n326 = event-data() -> ()  [unwired: 1 in, 5 out]
        n327 = local read "Travel per Pulse (mm)"() -> (w815:dbl)
        n328 = local read "1  Max"() -> (w820:dbl)
        n329 = local read "1 Rate"() -> (w819:dbl)
        n330 = local read "2 Rate"() -> (w816:dbl)
        n331 = local read "2 Max"() -> (w817:dbl)
        n332 = local read "1 Min"() -> (w821:dbl)
        n333 = local read "2 Min"() -> (w818:dbl)
        n334 = call "Sigma_SetSpeed.vi"("VISA resource name"=w826, "Travel per Pulse (0.004mm)"=w815, "Min (1mm) 2"=w818, "Max (2mm) 2"=w817, "Rate (1mm) 2"=w816, "error in (no error)"=w823, "Axis (1)"="W", "Min (1mm)"=w821, "Max (2mm)"=w820, "Rate (1mm)"=w819) -> ("VISA resource name out"=w825:refnum<visa-resource-name>, "error out"=w824:errorcluster)  [unwired: 8 in]
      }
      event "Right": Value Change {
        n335 = event-data() -> ()  [unwired: 1 in, 1 out]
        n336 = case shown="True" "Right" {
          tunnel: [w833 w839] -> w831
          tunnel: [w832 w838] -> w830
          tunnel: w829 -> [w833 w841]
          tunnel: w828 -> [w832 w840]
          frame False {
          }
          frame True {
            n337 = local read "Travel per Pulse (mm)"() -> (w835:dbl)
            n338 = local read "Move Distance"() -> (w834:dbl)
            n339 = call "Sigma_MoveAbs.vi"("Direction (+)"=FALSE, "Axis (1)"=1, "error in (no error)"=w840, "Travel (1mm)"=w834, "Travel per Pulse (0.004mm)"=w835, "VISA resource name"=w841) -> ("error out"=w838:errorcluster, "VISA resource name out"=w839:refnum<visa-resource-name>)  [unwired: 4 in]
          }
        }
      }
      event "Left": Value Change {
        n340 = event-data() -> ()  [unwired: 1 in, 1 out]
        n341 = case shown="True" "Left" {
          tunnel: [w848 w855] -> w846
          tunnel: [w847 w854] -> w845
          tunnel: w844 -> [w848 w856]
          tunnel: w843 -> [w847 w853]
          frame False {
          }
          frame True {
            n342 = local read "Travel per Pulse (mm)"() -> (w850:dbl)
            n343 = local read "Move Distance"() -> (w849:dbl)
            n344 = call "Sigma_MoveAbs.vi"("Direction (+)"=TRUE, "Axis (1)"=1, "error in (no error)"=w853, "Travel (1mm)"=w849, "Travel per Pulse (0.004mm)"=w850, "VISA resource name"=w856) -> ("error out"=w854:errorcluster, "VISA resource name out"=w855:refnum<visa-resource-name>)  [unwired: 4 in]
          }
        }
      }
      event "Front": Value Change {
        n345 = event-data() -> ()  [unwired: 1 in, 1 out]
        n346 = case shown="True" "Front" {
          tunnel: [w863 w869] -> w861
          tunnel: [w862 w868] -> w860
          tunnel: w859 -> [w863 w871]
          tunnel: w858 -> [w862 w870]
          frame False {
          }
          frame True {
            n347 = local read "Travel per Pulse (mm)"() -> (w865:dbl)
            n348 = local read "Move Distance"() -> (w864:dbl)
            n349 = call "Sigma_MoveAbs.vi"("Direction (+)"=FALSE, "Axis (1)"=2, "error in (no error)"=w870, "Travel (1mm)"=w864, "Travel per Pulse (0.004mm)"=w865, "VISA resource name"=w871) -> ("error out"=w868:errorcluster, "VISA resource name out"=w869:refnum<visa-resource-name>)  [unwired: 4 in]
          }
        }
      }
      event "Back": Value Change {
        n350 = event-data() -> ()  [unwired: 1 in, 1 out]
        n351 = case shown="True" "Back" {
          tunnel: [w878 w884] -> w876
          tunnel: [w877 w883] -> w875
          tunnel: w874 -> [w878 w886]
          tunnel: w873 -> [w877 w885]
          frame False {
          }
          frame True {
            n352 = local read "Travel per Pulse (mm)"() -> (w880:dbl)
            n353 = local read "Move Distance"() -> (w879:dbl)
            n354 = call "Sigma_MoveAbs.vi"("Direction (+)"=TRUE, "Axis (1)"=2, "error in (no error)"=w885, "Travel (1mm)"=w879, "Travel per Pulse (0.004mm)"=w880, "VISA resource name"=w886) -> ("error out"=w883:errorcluster, "VISA resource name out"=w884:refnum<visa-resource-name>)  [unwired: 4 in]
          }
        }
      }
      event "Home X": Value Change {
        n355 = event-data() -> ()  [unwired: 1 in, 1 out]
        n356 = case shown="True" "Home X" {
          tunnel: [w893 w896] -> w888
          tunnel: [w892 w895] -> w887
          tunnel: w891 -> [w893 w898]
          tunnel: w890 -> [w892 w897]
          frame False {
          }
          frame True {
            n357 = call "Sigma_Home.vi"("Axis (1)"="1", "error in (no error)"=w897, "VISA resource name"=w898) -> ("error out"=w895:errorcluster, "VISA resource name out"=w896:refnum<visa-resource-name>)  [unwired: 7 in]
          }
        }
      }
      event "Home Y": Value Change {
        n358 = event-data() -> ()  [unwired: 1 in, 1 out]
        n359 = case shown="True" "Home Y" {
          tunnel: [w905 w908] -> w901
          tunnel: [w904 w907] -> w900
          tunnel: w903 -> [w905 w910]
          tunnel: w902 -> [w904 w909]
          frame False {
          }
          frame True {
            n360 = call "Sigma_Home.vi"("Axis (1)"="2", "error in (no error)"=w909, "VISA resource name"=w910) -> ("error out"=w907:errorcluster, "VISA resource name out"=w908:refnum<visa-resource-name>)  [unwired: 7 in]
          }
        }
      }
      event "Stop 3": Value Change {
        n361 = event-data() -> ()  [unwired: 1 in, 1 out]
        n362 = case shown="True" "Stop 3" {
          tunnel: [w917 w918] -> w915
          tunnel: [w916 w919] -> w914
          tunnel: w913 -> [w917 w921]
          tunnel: w912 -> [w916 w920]
          frame False {
          }
          frame True {
            n363 = call "Sigma_Stop.vi"("Axis (1)"="W", "error in (no error)"=w920, "VISA resource name"=w921) -> ("error out"=w919:errorcluster, "VISA resource name out"=w918:refnum<visa-resource-name>)  [unwired: 7 in]
          }
        }
      }
      event "Emergency Stop": Value Change {
        n364 = event-data() -> ()  [unwired: 1 in, 1 out]
        n365 = case shown="True" "Emergency Stop" {
          tunnel: [w929 w932] -> w927
          tunnel: [w928 w931] -> w926
          tunnel: w925 -> [w929 w934]
          tunnel: w924 -> [w928 w933]
          frame False {
          }
          frame True {
            n366 = call "Sigma_Stop.vi"("Axis (1)"="E", "error in (no error)"=w933, "VISA resource name"=w934) -> ("error out"=w931:errorcluster, "VISA resource name out"=w932:refnum<visa-resource-name>)  [unwired: 7 in]
          }
        }
      }
    }
    n367 = Unbundle By Name(w772) -> ("status"=w773:bool)
    n368 = Compound Arithmetic op=OR(w773, w769) -> (w771:bool)
  }
  n369 = call <vilib>:"DAQmx Stop Task.vi"("task/channels in"=w25, "error in"=w26) -> ("task out"=w28:refnum<k21>, "error out"=w27:errorcluster)  [unwired: 12 in]
  n370 = call <vilib>:"DAQmx Clear Task.vi"("task in"=w28, "error in"=w27) -> ("error out"=w20:errorcluster)  [unwired: 13 in]
  n371 = call <vilib>:"Simple Error Handler.vi"("error in (no error)"=w20) -> ()  [unwired: 4 in, 5 out]
  n372 = VISA Close(VISA resource name=w38, error in (no error)=w39) -> (error out=w37:errorcluster)
  n373 = call <vilib>:"Simple Error Handler.vi"("error in (no error)"=w37) -> ()  [unwired: 4 in, 5 out]
  n374 = call <vilib>:"DAQmx Clear Task.vi"("task in"=w72, "error in"=w71) -> ("error out"=w80:errorcluster)  [unwired: 13 in]
  n375 = call <vilib>:"Simple Error Handler.vi"("error in (no error)"=w80) -> ()  [unwired: 4 in, 5 out]
  n376 = call <vilib>:"Simple Error Handler.vi"() -> ()  [unwired: 5 in, 5 out]
  "Move X" <- FALSE ("Move X")
